vi "WHD_VEten_0.1.1_Pruebas.vi"() -> ()   [LabVIEW 2015]
uses:
  <vilib>/LabVIEW Targets/FPGA/cRIO/shared/nicrio_ModuleControls/nicrio_cRIO-9234_DataRatesRing2.ctl
  <vilib>/RTwatchdog.llb/Watchdog expiration actions.ctl
  <vilib>/userdefined/High Color/nirio_resource_hc.ctl
  <vilib>/FPGAPlugInAG/cRIO-9031/niLvFpga_Open_cRIO-9031.vi
  <vilib>/Utility/file.llb/Write Delimited Spreadsheet (string).vi
  <vilib>/FPGAPlugInAG/cRIO-9031/niLvFpga_Run_cRIO-9031.vi
  <vilib>/Utility/error.llb/Error Cluster From Error Code.vi
  <vilib>/rvi/errors/niLvFpgaAdjustHostInterfaceError.vi
  <vilib>/rvi/interface/common/niFpgaWaitOnOcc.vi
  <vilib>/FPGAPlugInAG/cRIO-9031/niLvFpga_Reset_cRIO-9031.vi
  <vilib>/FPGAPlugInAG/cRIO-9031/niLvFpga_Close_cRIO-9031.vi
  <vilib>/rvi/interface/nirviOpenFPGA/nirviOpenFPGA.xnode
  FPGA Bitfiles/W&RDEuskotrenIBA_FPGATarget2_FPGA8a2wsBIdirec_MwruJOs6jio.lvbitx
  <vilib>/rvi/interface/nirviMethod/nirviMethod.xnode
  <vilib>/rvi/interface/nirviReadWriteControl/nirviReadWriteControl.xnode
  <vilib>/rvi/interface/nirviCloseFPGA/nirviCloseFPGA.xnode
  <vilib>/NI_Real-Time Target Support.lvlib
  NiFpgaLv.dll
  <vilib>/rvi/errors/niLvFpgaMergeErrorWithErrorCode.vi
  <vilib>/nisyscfg/nisyscfg.lvlib
  <vilib>/FPGAPlugInAG/cRIO-9031/niLvFpga_ConfigureFifo_cRIO-9031.vi
  <vilib>/FPGAPlugInAG/cRIO-9031/niLvFpga_StartFifo_cRIO-9031.vi
  <vilib>/FPGAPlugInAG/cRIO-9031/niLvFpga_ReadFifo_cRIO-9031.vi
  <vilib>/FPGAPlugInAG/cRIO-9031/niLvFpga_StopFifo_cRIO-9031.vi
  AURA_Wheel/Json2Labv.lvlib
  AURA_Wheel/AuraWheelAPI/AuraWheel.lvlib
panel:
  in  "stop":bool
  out "Direccion 0?":bool
  out "Boton Adquirir?":bool
  out "RuedaDetectada2?":bool=TRUE
  out "RuedaDetectada1?":bool=TRUE
  in  "Timeout ruedas":dbl
  in  "Borrar archivos\nadquisicion con error":bool
  in  "Disable watchdog?":bool
  in  "Reset watchdog?":bool
  in  "Leer config RFID NEM":bool
  in  "bytes to read":i32
  in  "DeviceAddress":u8
  in  "timeout ms (60000)":i32
  in  "Max archivos":u32=2
  in  "Bytes libre despues de borrar":u32=2
  in  "Bytes min libre":u32=2
  in  "Nº de acelerómetros":i32
  in  "Nº inductivos":i32
  in  "Offset_rueda WS 1":fxp<+/-,24,-4>=0.004999998956918716 format="%.27g"
  out "TAGs_AURAwheel":string[][](array[string])
  out "Plataformas?":bool
  out "Nº Ejes":i32[](array[numeric])
  out "Nº UTs":i32
  out "it-read-LR6":i32[](array[numeric])
  out "it-LR6":i32
  out "RFID_LR6_Error":errorcluster
  out "Series_flota":string[](array[string])
  out "Tabla_flota":string[][](array[string])
  out "Puntos medios de las ventanas":dbl[][](array[numeric])
  out "configuration file path":path=path "c:/Parametros.cfg"
  in  "IP synchr":string
  out "data":cluster{"status":string}
  out "confRFID":path=path "c:/RFID/TAGS.csv"
  out "TAGS leidos":path=path "c:/RFID/TAGS.csv"
  in  "Use Aura?":bool
  in  "Parametros AuraWheel":string[](array[string])
  in  "Parámetros acelerómetros":dbl[](array[numeric])
  in  "Tiempo de adquisicion":dbl=10.0
  in  "Adquirir":bool
  out "Fin":bool
  out "Contador":i32=1
  out "Path TEST":path=path "c:/TEST"
  out "Fallo fotocelula":bool
  out "Path_Borrar":path=path "c:/Trenes"
  out "Longitud de la unidad":dbl
  out "Aviso no detección":string
  out "Time to Acquire Block (ms)":i32
  out "Distancia de acelerómetros":dbl[](array[numeric])
  out "Block Size":u32
  out "Distancias generales":dbl[](array[numeric])
  in  "Reset del controlador":bool
  in  "Configuración":bool
  in  "Parar la aplicación":bool
  out "RFID":bool=TRUE
  out "date/time string":string
  out "Timeout ruedas":bool
  out "Tiempo":dbl
  out "Inicio pasada":timestamp
  out "Ultimo TEST":timestamp
  out "Fuente":bool=TRUE
  out "Estado":string
  out "RFID_ID":refnum<k5>
  out "DC OK":string
  out "Aviso temperatura":string
  in  "Tab Control":T1(tab)=enum."Parámetros"
  out "V (m/s)":dbl
  out "Temperatura (ºC)":dbl
  out "Max RMS Ruedas":dbl[][](array[numeric])
  out "result":bool
  out "TAGs":string[](array[string])
  out "Parar":bool
  out "TAGs LR6":string[](array[string])
  out "TAGs HEX":string[](array[string])
  out "Waveform Graph":sgl[][](graph)
  out "Nombre de archivo":path[](array[path])
  out "Tiempo de paso (s)":dbl
  out "Tiempo extra de adquisición (s)":dbl
  out "Número de ejes detectados":i32
  out "Buffer Underflow":bool
  out "Buffer Overflow":bool
  out "created path":path
  out "Nº Ruedas 1":i32
  out "NºRuedas 2":i32
  out "deleted portion":sgl[](array[numeric])
  out "deleted portion 2":sgl[](array[numeric])
  out "Ejes_convoy":i32
  out "T fuera rango":bool
  in  "Frecuencia de muestreo (Hz)":dbl=25600.0
  in  "Escaneos de la FIFO por canal":u32=5000
  in  "Tiempo extra al detector de paso (s)":dbl=1.0
  in  "dt RMS":dbl=256.0
  in  "Frecuencia de muestreo y módulo CRIO":T2=2 items=["51.200 kS/s (NI 9234)"=1, "25.600 kS/s (NI 9234)"=2, "17.067 kS/s (NI 9234)"=3, "12.800 kS/s (NI 9234)"=4, "10.240 kS/s (NI 9234)"=5, "8.533 kS/s (NI 9234)"=6, "7.314 kS/s (NI 9234)"=7, "6.400 kS/s (NI 9234)"=8, "5.689 kS/s (NI 9234)"=9, "5.120 kS/s (NI 9234)"=10, "4.654 kS/s (NI 9234)"=11, "4.267 kS/s (NI 9234)"=12, "3.938 kS/s (NI 9234)"=13, "3.657 kS/s (NI 9234)"=14, "3.413 kS/s (NI 9234)"=15, "3.200 kS/s (NI 9234)"=16, "3.012 kS/s (NI 9234)"=17, "2.845 kS/s (NI 9234)"=18, "2.695 kS/s (NI 9234)"=19, "2.560 kS/s (NI 9234)"=20, "2.438 kS/s (NI 9234)"=21, "2.328 kS/s (NI 9234)"=22, "2.226 kS/s (NI 9234)"=23, "2.133 kS/s (NI 9234)"=24, "2.048 kS/s (NI 9234)"=25, "1.969 kS/s (NI 9234)"=26, "1.896 kS/s (NI 9234)"=27, "1.829 kS/s (NI 9234)"=28, "1.765 kS/s (NI 9234)"=29, "1.707 kS/s (NI 9234)"=30, "1.652 kS/s (NI 9234)"=31]
  in  "Puerto RFID":u16=2189
  in  "IP RFID":string="192.168.106.99"
  in  "Offset_rueda WS 2":fxp<+/-,24,-4>=0.004999998956918716 format="%.27g"
  in  "Count(mSec)":u32=2
  in  "LR6 IP address":string="192.168.106.94"
  in  "Port LR6":u16=2001
  in  "RFID NEM on?":bool
  in  "RFID LR6 on?":bool
  in  "Canal cero WS1?":bool
  in  "Canal cero WS2":bool
  out "Parámetros":bool=TRUE
  out "Distacias y medidas de dispositivos":bool=TRUE
  out "RFID_Error":errorcluster
  out "error FPGA":errorcluster
  out "error manipulacion archivos":errorcluster
  out "Unidades y ejes":bool=TRUE
  out "RFID":bool=TRUE
  out "error AURA":errorcluster
  out "Response headers":string
  in  "Array":path[](array[path])=[path "c:/Trenes_prueba/0207_2013-09-24_19-09-42_0.bin", path "c:/Trenes_prueba/0096_2013-10-30_18-13-14_0.bin", path "c:/Trenes_prueba/0001_2013-06-05_13-06-23_0.bin"]
  out "Numeric 3":i32
  in  "Digital?":bool=TRUE
  out "Bucle Espera":i32
  out "Watchdog config":T3={"reset"=FALSE, "occurrence"=FALSE, "trigger protocol"=enum."active high", "trigger line"=enum."none", "disable watchdog on VI exit"=TRUE}
  # "Funciona?"
  # "Última detección de unidad"
  # "Error!!"
  # "Estado de la memoria"
  # "Parámetros de muestreo"
  # "Parámetros de adquisición"
  # "Parámetros de procesado"
  # "Cambio Fecha y Hora"
  # "Cargar datos de configuración"
  # "Errores!!"
  # "WRD_MEX\nWRD_ZAR"
  # "0 tagMexInit\n1 tagMexFin\n\n0 tag1\n1 tag2"
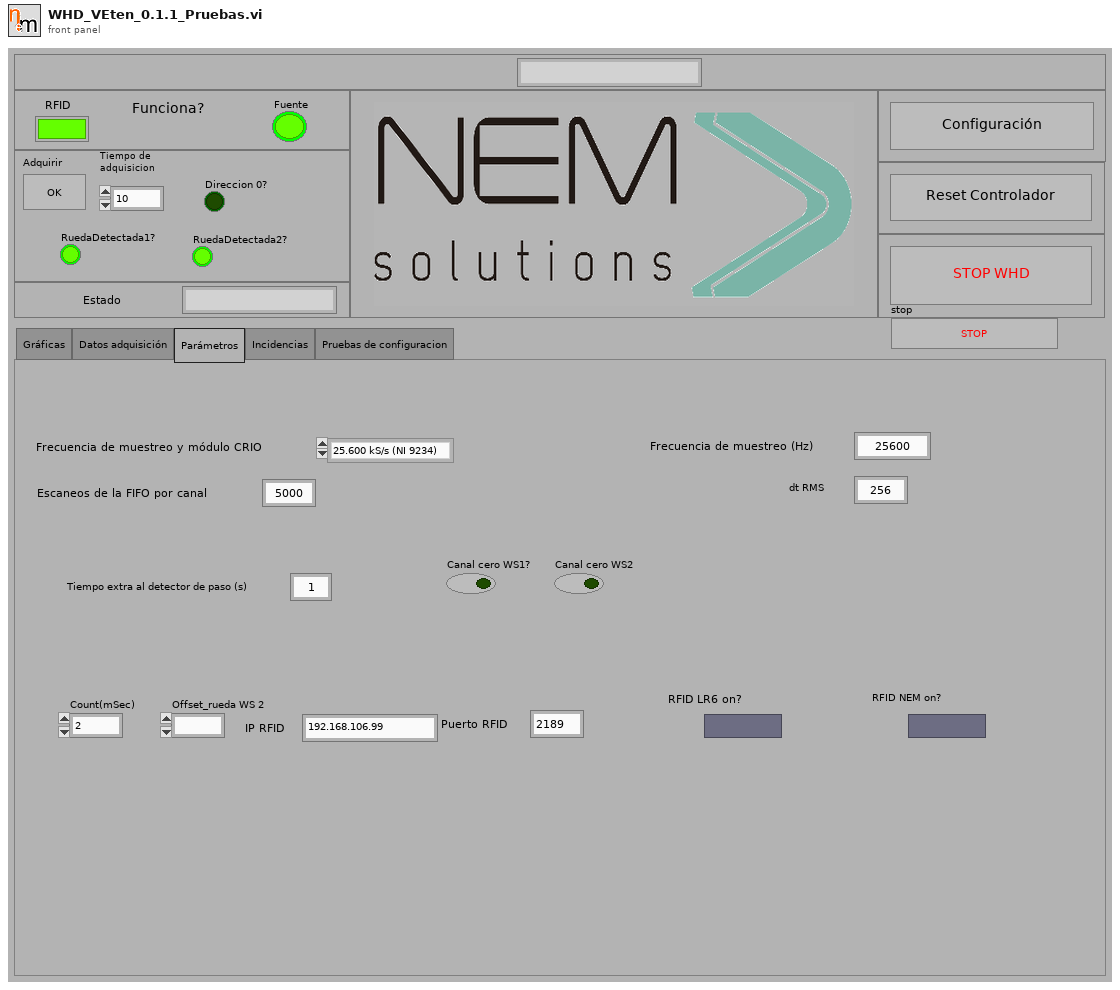
[diagram p1: front panel]
types:
  T1 = enum32{"Gráficas", "Datos adquisición", "Parámetros", "Incidencias", "Pruebas de configuracion"}
  T2 = typedef "nicrio_cRIO-9234_DataRatesRing2.ctl" = u8
  T3 = typedef "Watchdog expiration actions.ctl" = cluster{"reset":bool, "occurrence":bool, "trigger protocol":enum16{"active high", "active low", "open collector"}, "trigger line":enum16{"none", "line 0", "line 1", "line 2", "line 3", "line 4", "line 5", "line 6", "line 7", "SMB line 0"}, "disable watchdog on VI exit":bool}
  T4 = typedef "nirio_resource_hc.ctl" = tag
  T5 = enum16{"Standard", "Buffered", "CRLF", "Immediate"}
  T6 = enum16{"open", "replace", "create", "open or create", "replace or create", "replace or create with confirmation"}
  T7 = enum16{"big-endian, network order", "native, host order", "little-endian"}
  T8 = cluster{"error IO":errorcluster, bool[], u32[], string[], dbl[]}
  T9 = cluster{"g_ts":dbl, "p_sp":dbl, "p_tp":dbl, "p_tg":cluster{"tg_n":dbl, "tg_t":string}[], "p_ax":cluster{"ax_n":dbl, "ax_sp":dbl, "ax_wh":cluster{"wh_p":dbl, "wh_a1":dbl, "wh_a2":dbl, "wh_a3":dbl, "wh_a4":dbl}[]}[]}
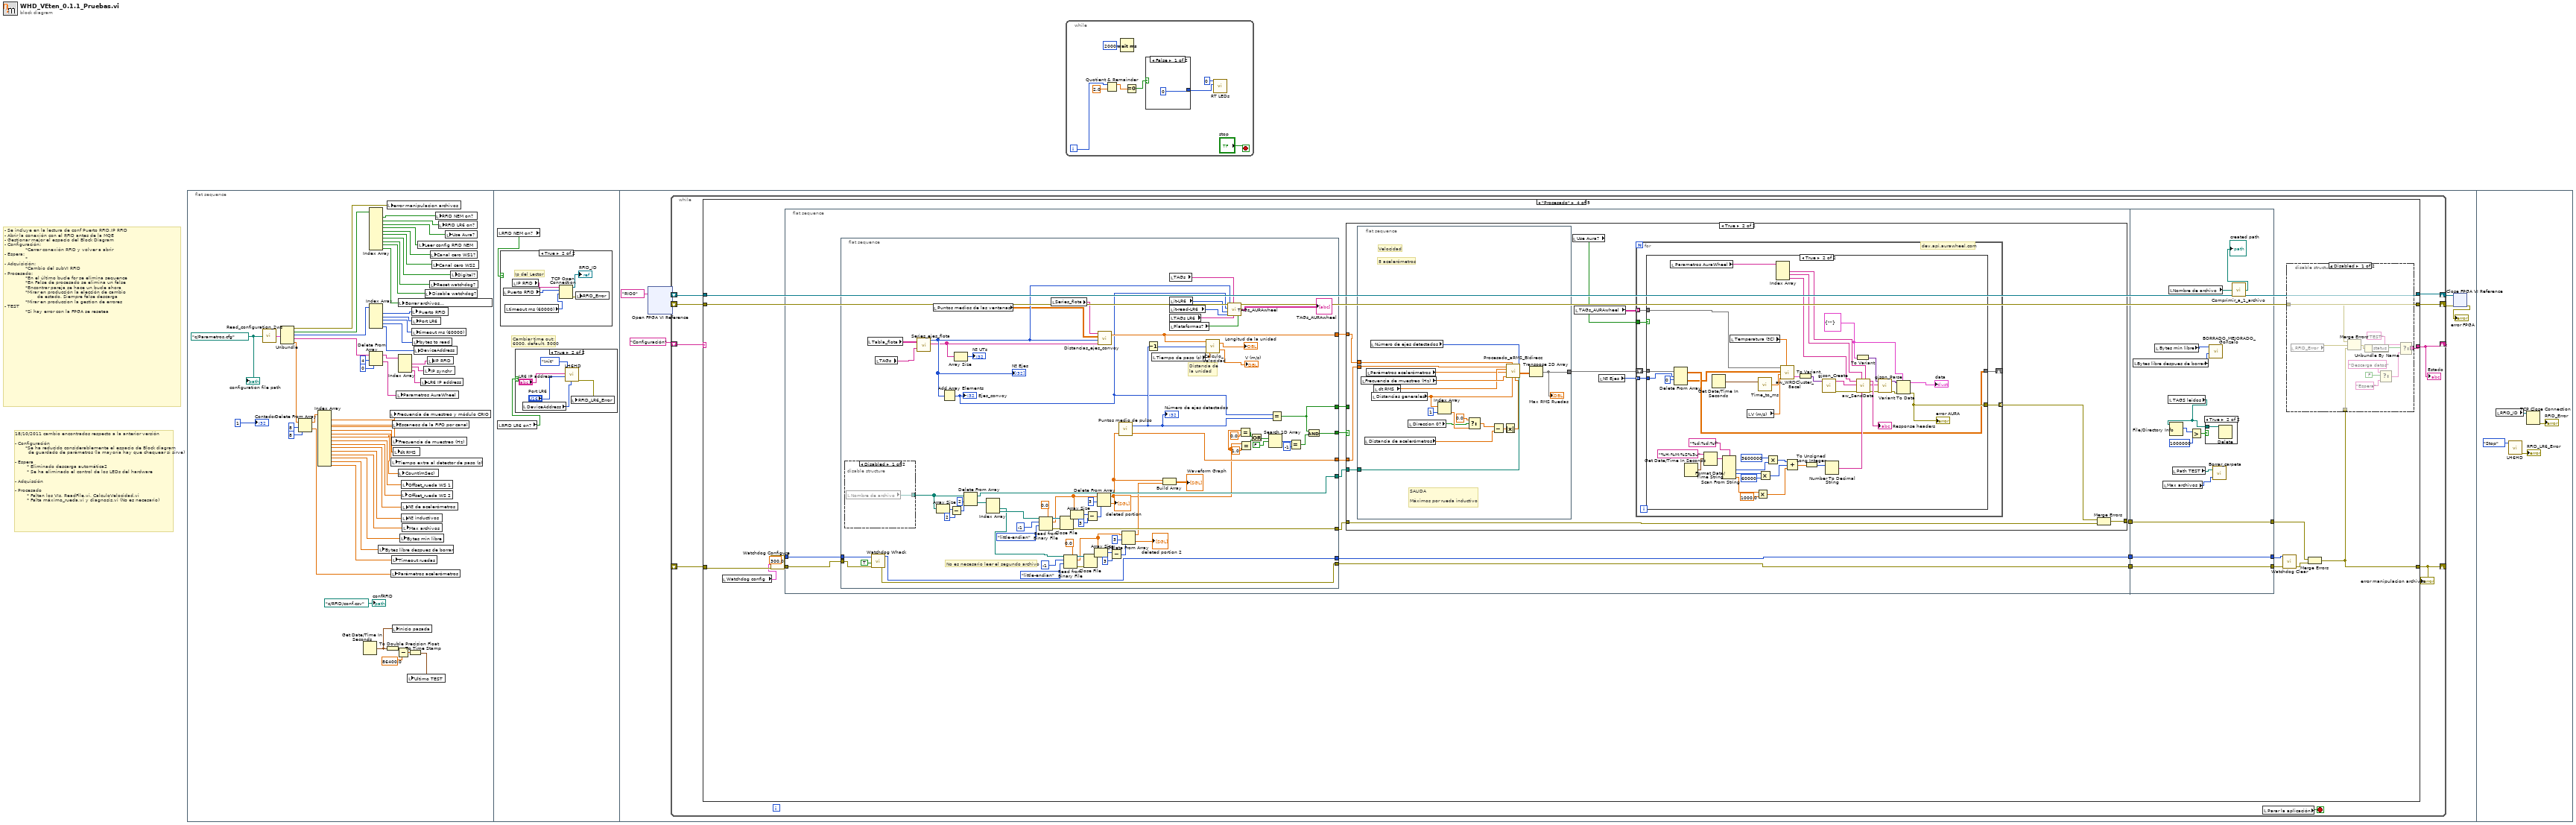
[diagram p0: block diagram]
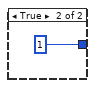
[diagram p2: hidden frame]
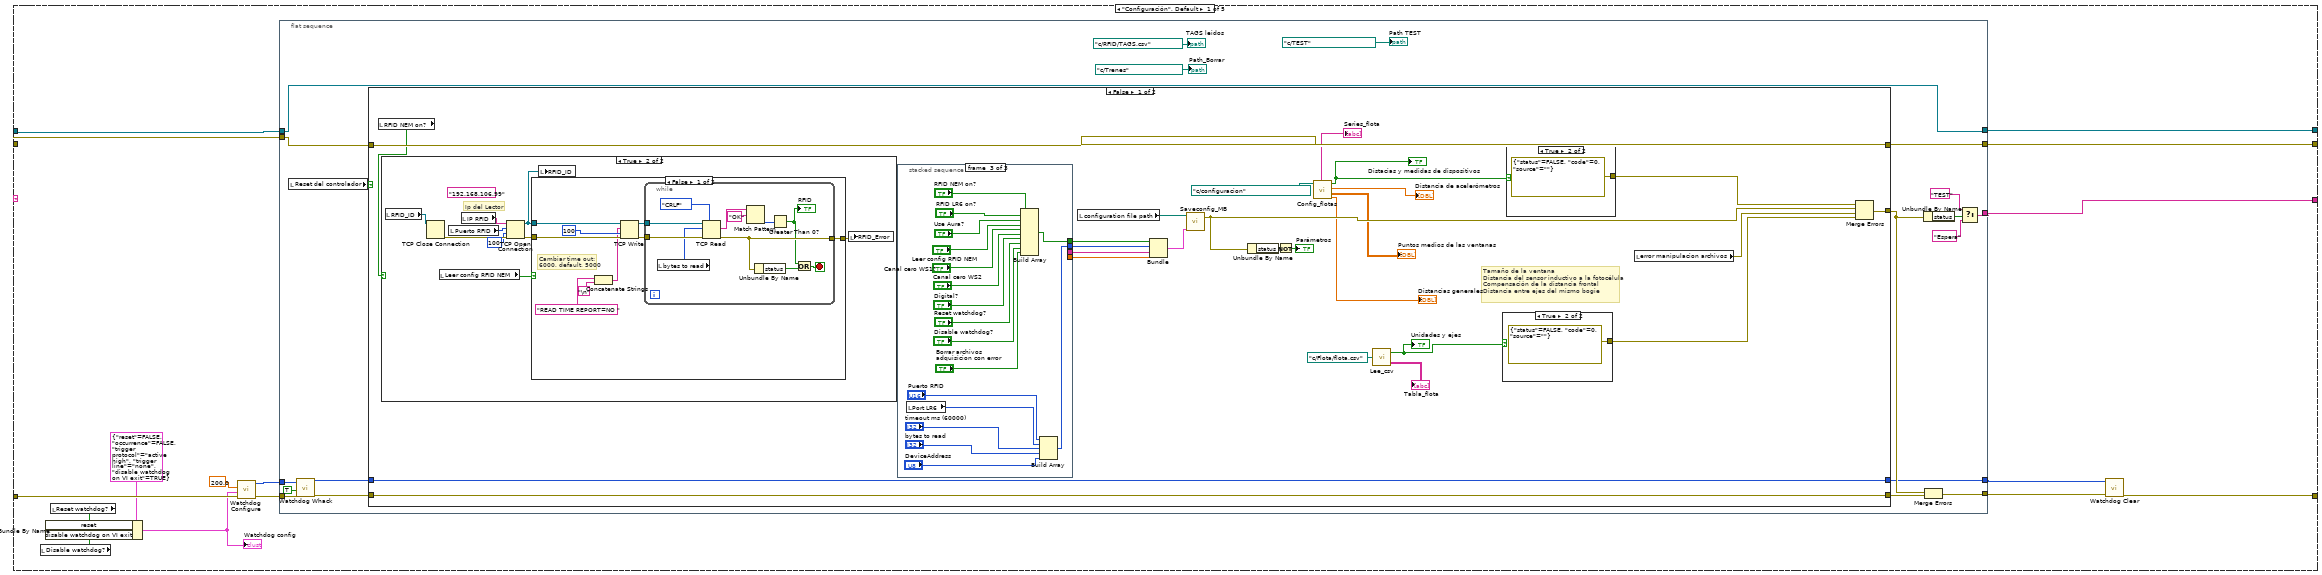
[diagram p5: hidden frame]
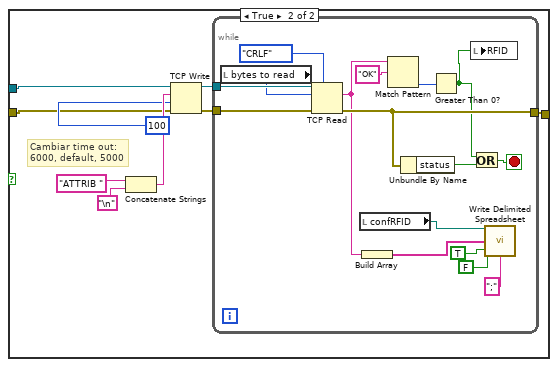
[diagram p7: hidden frame]
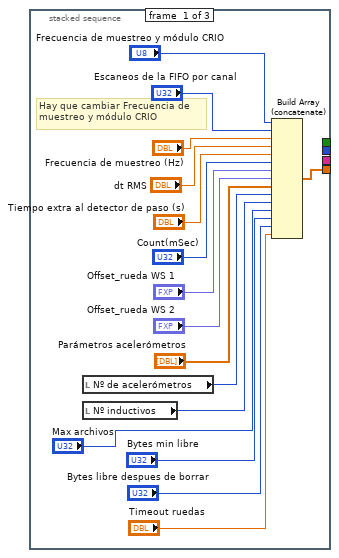
[diagram p8: hidden frame]
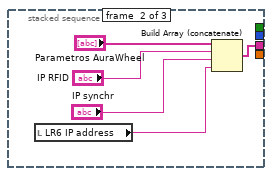
[diagram p9: hidden frame]
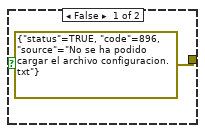
[diagram p10: hidden frame]
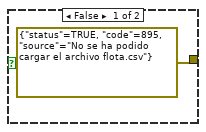
[diagram p11: hidden frame]
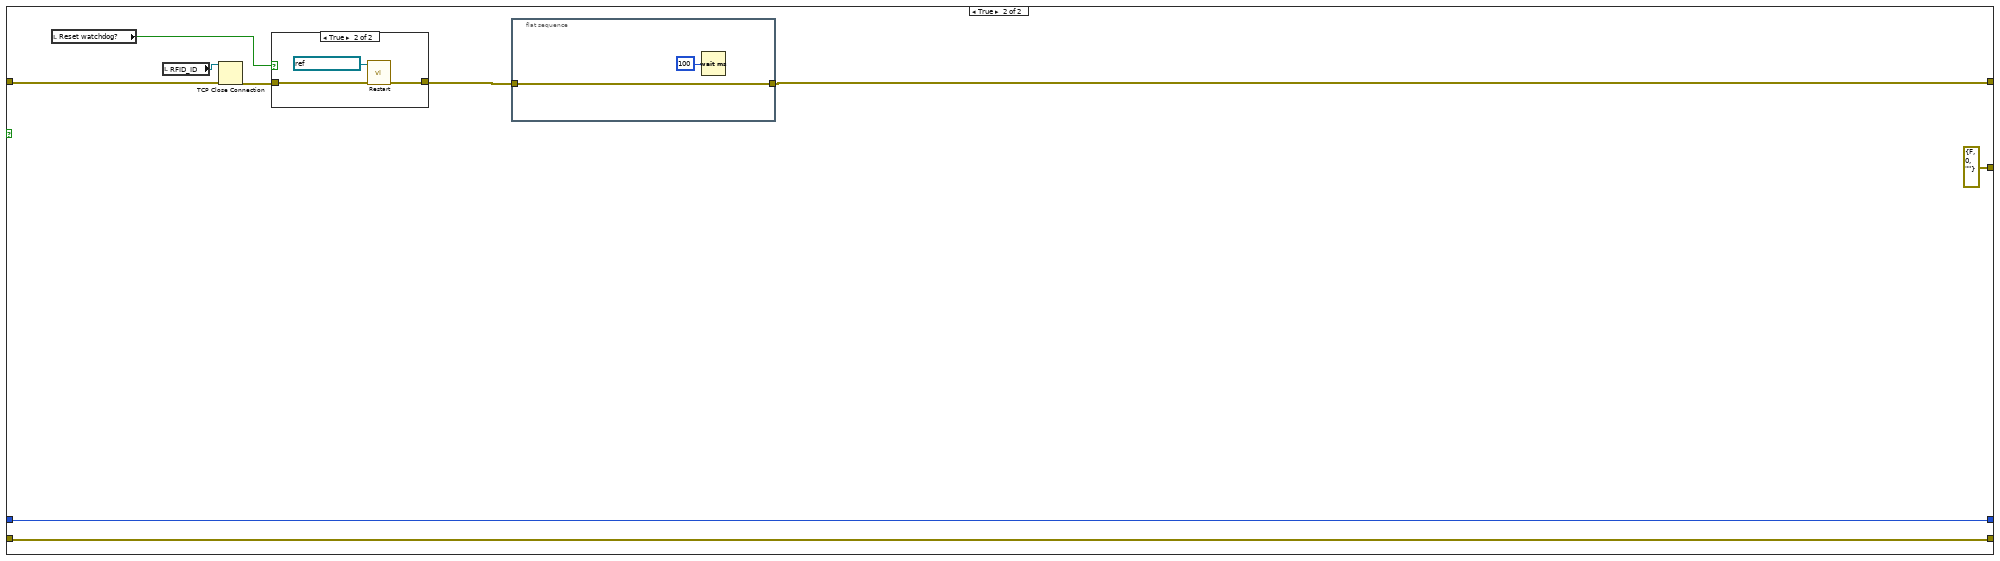
[diagram p12: hidden frame]
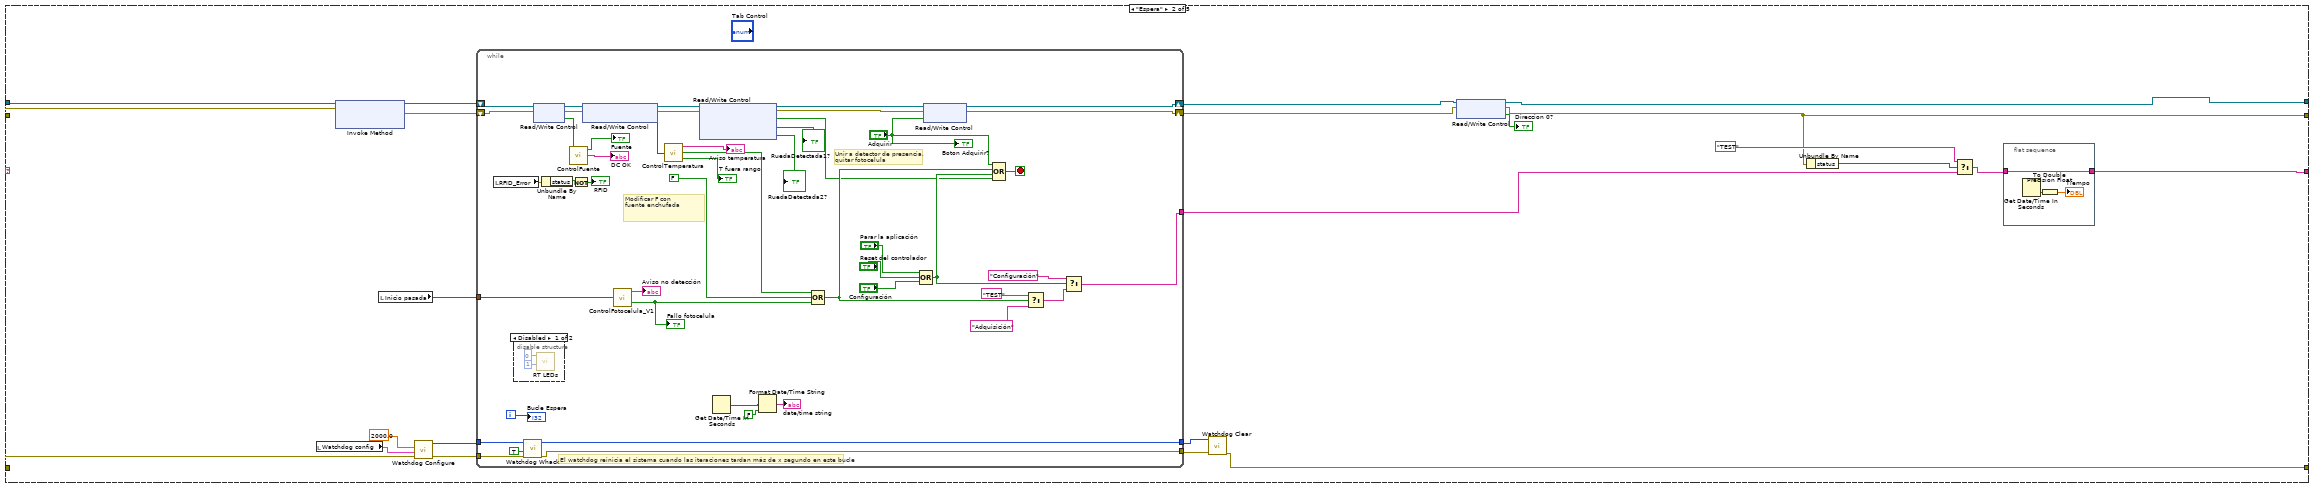
[diagram p14: hidden frame]
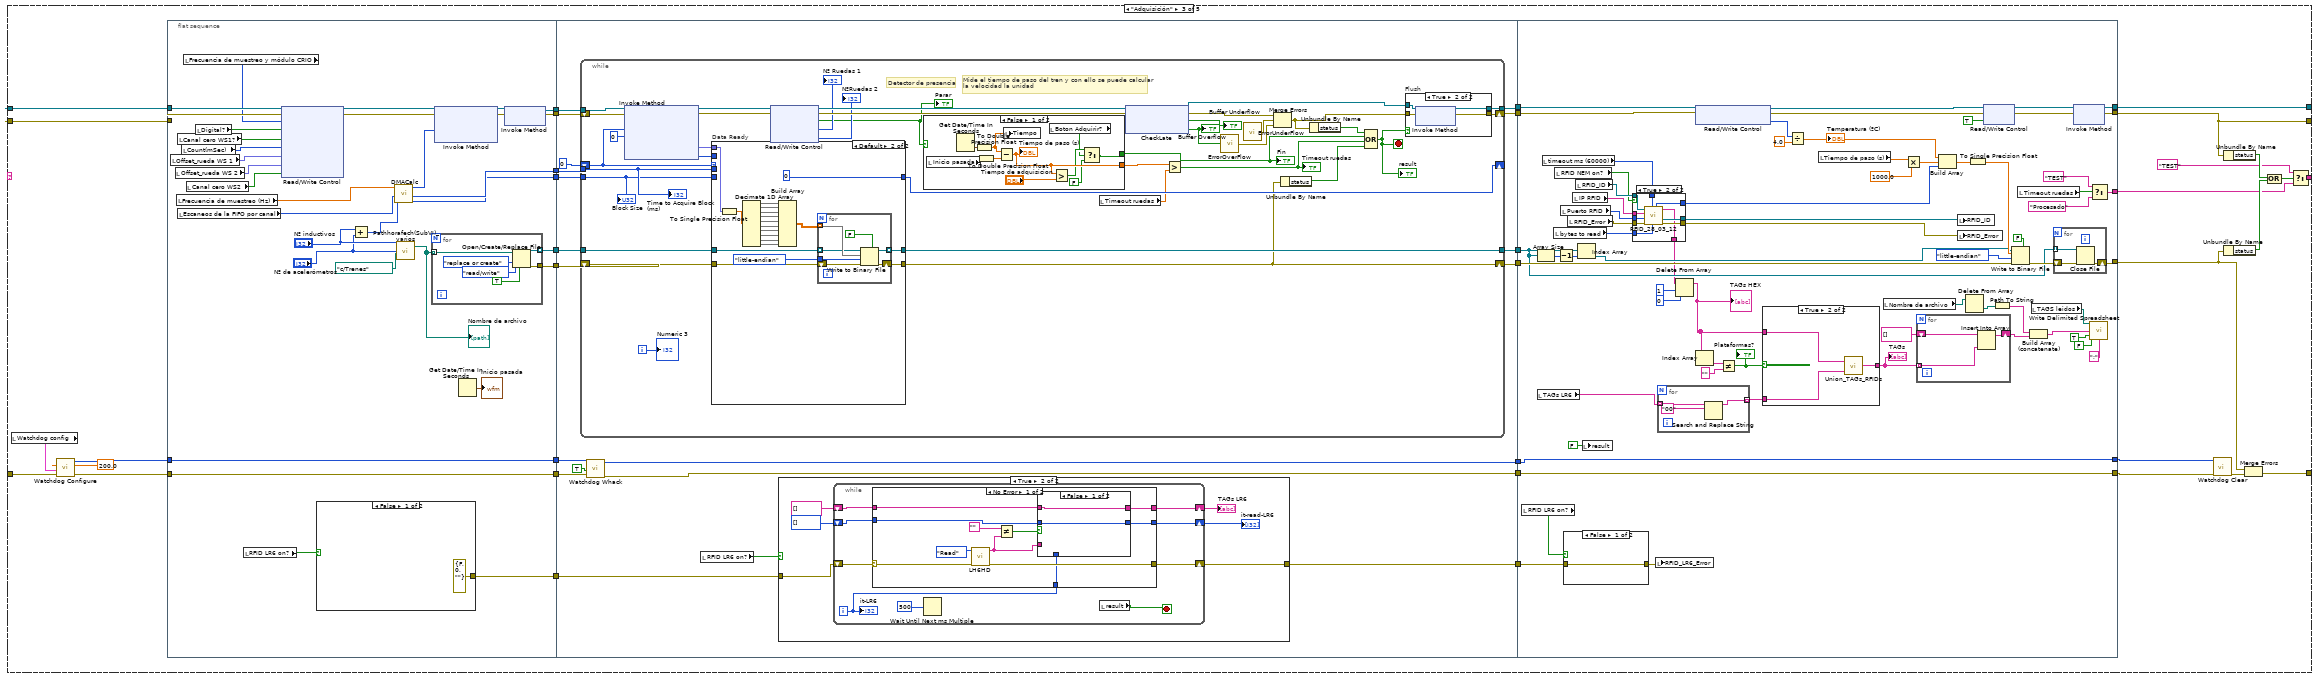
[diagram p16: hidden frame]
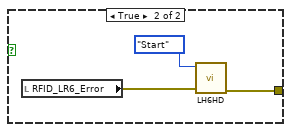
[diagram p17: hidden frame]
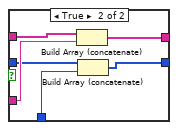
[diagram p19: hidden frame]
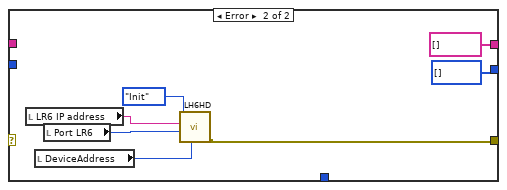
[diagram p20: hidden frame]
diagram:
  # "18/10/2011 cambio encontrados respecto a la anterior versión\n\n- Configuración\n       *Se ha reducido considerablemente el espacio de Block diagram\n         de guardado de parámetros (la mayoría hay que chequear si sirve)\n\n- Espera\n        * Eliminado descarga automática2\n        * Se ha eliminado el control de los LEDs del hardware\n       \n- Adquisción\n\n- Procesado\n        * Faltan los VIs, ReadFile.vi, CalculoVelocidad.vi\n        * Falta máximo_rueda.vi y diagnosis.vi (No es necesario)"
  # "- Se incluye en la lectura de conf Puerto RFID,IP RFID\n- Abrir la conexión con el RFID antes de la MQE\n- Gestionar mejor el espacio del Block Diagram\n- Configuración:\n              *Cerrar conexión RFID y volver a abrir\n- Espera:\n              *\n- Adquisición:\n              *Cambio del subVI RFID\n- Procesado:\n              *En el último bucle for se elimina sequence\n              *En False de procesado se elimina un false\n              *Encontrar pareja se hace un bucle ahora\n              *Mirar en producción la elección de cambio\n                      de estado. Siempre false descarga \n              *Mirar en produccion la gestion de errores\n- TEST\n              *Si hay error con la FPGA se resetea"
  n1 = flat-sequence {
    frame #0 {
      w38 = path "c:/Parametros.cfg" ("configuration file path")
      n2 = call "Read_configuration_2ws.vi"("configuration file path"=w38) -> ("output cluster"=w37:T8)
      n3 = Unbundle(w37) -> ("error IO"=w42:errorcluster, w41:bool[], w40:u32[], w29:string[], w35:dbl[])
      n4 = Delete From Array(array=w35, length=8, index=8) -> (deleted portion=w31:dbl[], array with subset deleted=w34:dbl[])
      n5 = Index Array(array=w34) -> (element #1=w49:dbl, element #2=w48:dbl, element #3=w47:dbl, element #4=w46:dbl, element #5=w45:dbl, element #6=w18:dbl, element #7=w17:dbl, element #8=w24:dbl, element #9=w16:dbl, element #10=w15:dbl, element #11=w14:dbl, element #12=w13:dbl, element #13=w12:dbl, element #14=w1:dbl)  [unwired: 14 in]
      n6 = Get Date/Time In Seconds() -> (seconds since 1Jan1904=w51:timestamp)
      n7 = Index Array(array=w41) -> (element #1=w44:bool, element #2=w43:bool, element #3=w30:bool, element #4=w8:bool, element #5=w7:bool, element #6=w6:bool, element #7=w5:bool, element #8=w4:bool, element #9=w3:bool, element #10=w2:bool)  [unwired: 10 in]
      n8 = Index Array(array=w40) -> (element #1=w36:u32, element #2=w19:u32, element #3=w11:u32, element #4=w10:u32, element #5=w9:u32)  [unwired: 5 in]
      n9 = Delete From Array(array=w29, length=4, index=0) -> (deleted portion=w22:string[], array with subset deleted=w28:string[])
      n10 = local write "Bytes libre despues de borrar"(w12) -> ()
      n11 = To Double Precision Float(number=w51) -> (double precision float=w53:dbl)
      n12 = local write "error manipulacion archivos"(w42) -> ()
      n13 = local write "Frecuencia de muestreo y módulo CRIO"(w49) -> ()
      n14 = local write "Parámetros acelerómetros"(w31) -> ()
      n15 = local write "Tiempo extra al detector de paso (s)"(w45) -> ()
      n16 = local write "Frecuencia de muestreo (Hz)"(w47) -> ()
      n17 = local write "Timeout ruedas"(w1) -> ()
      n18 = local write "Escaneos de la FIFO por canal"(w48) -> ()
      n19 = local write "Inicio pasada"(w51) -> ()
      n20 = local write "dt RMS"(w46) -> ()
      n21 = local write "Parametros AuraWheel"(w22) -> ()
      n22 = Subtract(x=w53, y=86400.0) -> (x-y=w52:dbl)
      n23 = local write "Borrar archivos\nadquisicion con error"(w2) -> ()
      n24 = Index Array(array=w28) -> (element #1=w21:string, element #2=w23:string, element #3=w20:string)  [unwired: 3 in]
      n25 = local write "Count(mSec)"(w18) -> ()
      n26 = local write "Bytes min libre"(w13) -> ()
      n27 = local write "Offset_rueda WS 2"(w24) -> ()
      n28 = local write "Offset_rueda WS 1"(w17) -> ()
      n29 = local write "Nº de acelerómetros"(w16) -> ()
      n30 = local write "Nº inductivos"(w15) -> ()
      n31 = local write "Max archivos"(w14) -> ()
      n32 = To Time Stamp(1:w52) -> (0:w50:timestamp)
      n33 = local write "Ultimo TEST"(w50) -> ()
      n34 = local write "Puerto RFID"(w36) -> ()
      n35 = local write "Port LR6"(w19) -> ()
      n36 = local write "timeout ms (60000)"(w11) -> ()
      n37 = local write "bytes to read"(w10) -> ()
      n38 = local write "DeviceAddress"(w9) -> ()
      n39 = local write "Leer config RFID NEM"(w8) -> ()
      n40 = local write "LR6 IP address"(w20) -> ()
      n41 = local write "IP synchr"(w23) -> ()
      n42 = local write "Disable watchdog?"(w3) -> ()
      n43 = local write "IP RFID"(w21) -> ()
      n44 = local write "Reset watchdog?"(w4) -> ()
      n45 = local write "Canal cero WS1?"(w7) -> ()
      n46 = local write "Canal cero WS2"(w6) -> ()
      n47 = local write "RFID NEM on?"(w44) -> ()
      n48 = local write "RFID LR6 on?"(w43) -> ()
      n49 = local write "Use Aura?"(w30) -> ()
      n50 = local write "Digital?"(w5) -> ()
      "Contador" <- 1
      "confRFID" <- path "c:/RFID/conf.csv" ("file path (use dialog)")
      "configuration file path" <- w38
    }
    frame #1 {
      # "Cambiar time out:\n6000, default, 5000"
      n51 = local read "RFID NEM on?"() -> (w56:bool)
      n52 = local read "RFID LR6 on?"() -> (w55:bool)
      n53 = case shown="True" w56 {
        frame False {
        }
        frame True {
          # "Ip del Lector"
          n54 = local read "Puerto RFID"() -> (w64:u16)
          n55 = local read "timeout ms (60000)"() -> (w62:i32)
          n56 = local read "IP RFID"() -> (w65:string)
          n57 = TCP Open Connection(address=w65, remote port or service name=w64, timeout ms (60000)=w62) -> (connection ID=→"RFID_ID":refnum<k5>, error out=w63:errorcluster)  [unwired: 1 in, 1 out]
          n58 = local write "RFID_Error"(w63) -> ()
        }
      }
      n59 = case shown="True" w55 {
        frame False {
        }
        frame True {
          n60 = local read "DeviceAddress"() -> (w57:u8)
          n61 = call "LH6HD.vi"("DeviceAddress"=w57, "Reader Port"="Port LR6", "IP Address"="LR6 IP address", "Action"=enum16{"Init", "Start", "Read", "Stop", "Exit"}."Init") -> ("error out"=w61:errorcluster)  [unwired: 6 in, 1 out]
          n62 = local write "RFID_LR6_Error"(w61) -> ()
        }
      }
    }
    frame #2 {
      n63 = xnode "Open FPGA VI Reference"("resource name"=T4 "RIO0") -> ("FPGA VI Reference Out"=w73:refnum<k20>, "error out"=w72:errorcluster)  [unwired: 1 in]
      n64 = while {
        shift-right: [w77] -> _
        shift-left: "Configuración" -> [w82]
        shift-right: [w75] -> w69
        shift-left: w73 -> [w81]
        shift-right: [w74] -> w68
        shift-left: w72 -> [w80]
        shift-right: [w79] -> _
        shift-left: _ -> [w78]
        stop <- w76 stop-if-true
        n65 = case shown="\"Procesado\"" w82 {
          tunnel: [w97 w269 w345 w677 w910] -> w77
          tunnel: [w96 w257 w359 w679 w909] -> w75
          tunnel: [w98 w256 w360 w674 w907] -> w74
          tunnel: w81 -> [w95 w274 w367 w679 w909]
          tunnel: w80 -> [w94 w272 w366 w674 w908]
          tunnel: [w87 w263 w357 w676 w897] -> w79
          tunnel: w78 -> [w93 w268 w341 w673 w902]
          frame "Configuración", Default {
            n66 = local read "Disable watchdog?"() -> (w85:bool)
            n67 = local read "Reset watchdog?"() -> (w84:bool)
            n68 = Bundle By Name(cluster=T3 {"reset"=FALSE, "occurrence"=FALSE, "trigger protocol"=enum."active high", "trigger line"=enum."none", "disable watchdog on VI exit"=TRUE} ("expiration actions"), "reset"=w84, "disable watchdog on VI exit"=w85) -> (w83:T3)
            "Watchdog config" <- w83
            n69 = call <vilib>:"Watchdog Configure.vi"("error in (no error)"=w93, "expiration actions"=w83, "timeout (1 sec)"=200.0) -> ("error out"=w90:errorcluster, "watchdogID"=w91:u64)  [unwired: 3 in, 2 out]
            n70 = flat-sequence {
              tunnel: [w109] -> w98
              tunnel: [w117] -> w97
              tunnel: w95 -> [w110]
              tunnel: [w110] -> w96
              tunnel: [w112] -> w88
              tunnel: w94 -> [w107]
              tunnel: w91 -> [w105]
              tunnel: w90 -> [w104]
              tunnel: [w102] -> w89
              frame #0 {
                n71 = local read "Reset del controlador"() -> (w106:bool)
                n72 = call <vilib>:"Watchdog Whack.vi"("error in (no error)"=w104, "reset watchdog after expire? (F)"=TRUE, "watchdogID in"=w105) -> ("error out"=w100:errorcluster, "watchdogID out"=w101:u64)  [unwired: 2 in, 1 out]
                n73 = case shown="False" w106 {
                  tunnel: w107 -> [w144 w247]
                  tunnel: [w144 w246] -> w109
                  tunnel: [w130 errorcluster {"status"=FALSE, "code"=0, "source"=""} ("error IO")] -> w108
                  tunnel: [w122 w245] -> w102
                  tunnel: w101 -> [w122 w245]
                  tunnel: w100 -> [w121 w244]
                  tunnel: [w121 w244] -> w99
                  frame False {
                    # "Tamaño de la ventana\nDistancia del sensor inductivo a la fotocélula\nCompensación de la distancia frontal\nDistancia entre ejes del mismo bogie"
                    n74 = local read "RFID NEM on?"() -> (w120:bool)
                    n75 = case shown="True" w120 {
                      frame False {
                      }
                      frame True {
                        (unwired) "192.168.106.99" ("address")
                        # "Ip del Lector"
                        n76 = local read "RFID_ID"() -> (w152:refnum<k5>)
                        n77 = TCP Close Connection(connection ID=w152) -> (error out=w153:errorcluster)  [unwired: 2 in, 1 out]
                        n78 = local read "Leer config RFID NEM"() -> (w145:bool)
                        n79 = local read "Puerto RFID"() -> (w150:u16)
                        n80 = local read "IP RFID"() -> (w149:string)
                        n81 = TCP Open Connection(address=w149, remote port or service name=w150, timeout ms (60000)=100, error in (no error)=w153) -> (connection ID=w151:refnum<k5>, error out=w146:errorcluster)  [unwired: 1 out]
                        n82 = case shown="False" w145 {
                          tunnel: w151 -> [w162 w176]
                          tunnel: [w160 w174] -> w147
                          tunnel: w146 -> [w157 w175]
                          frame False {
                            # "Cambiar time out:\n6000, default, 5000"
                            n83 = Concatenate Strings("READ TIME REPORT=NO " ("data in"), "\n") -> (w154:string)
                            n84 = TCP Write(connection ID=w162, data in=w154, error in (no error)=w157, 9:100 ("timeout ms (25000)")) -> (connection ID out=w158:refnum<k5>, error out=w159:errorcluster)  [unwired: 1 out]
                            n85 = while {
                              tunnel: w159 -> [w172]
                              tunnel: w158 -> [w171]
                              tunnel: [w170] -> w160
                              stop <- w167 stop-if-true
                              n86 = local read "bytes to read"() -> (w163:i32)
                              n87 = TCP Read(connection ID=w171, bytes to read=w163, error in (no error)=w172, 7:T5."CRLF" ("mode (standard)")) -> (data out=w165:string, error out=w170:errorcluster)  [unwired: 1 in, 1 out]
                              n88 = Match Pattern(string=w165, regular expression="OK") -> (offset past match=w168:i32)  [unwired: 4 out]
                              n89 = Unbundle By Name(w170) -> ("status"=w166:bool)
                              n90 = Greater Than 0?(x=w168) -> (x > 0?=w164:bool)
                              "RFID" <- w164
                              n91 = Or(x=w164, y=w166) -> (x .or. y?=w167:bool)
                            }
                          }
                          frame True {
                            # "Cambiar time out:\n6000, default, 5000"
                            n92 = Concatenate Strings("ATTRIB " ("data in"), "\n") -> (w182:string)
                            n93 = TCP Write(connection ID=w176, data in=w182, error in (no error)=w175, 9:100 ("timeout ms (25000)")) -> (connection ID out=w179:refnum<k5>, error out=w178:errorcluster)  [unwired: 1 out]
                            n94 = while {
                              tunnel: w178 -> [w197]
                              tunnel: w179 -> [w196]
                              tunnel: [w195] -> w174
                              stop <- w192 stop-if-true
                              n95 = local read "bytes to read"() -> (w183:i32)
                              n96 = TCP Read(connection ID=w196, bytes to read=w183, error in (no error)=w197, 7:T5."CRLF" ("mode (standard)")) -> (data out=w186:string, error out=w195:errorcluster)  [unwired: 1 in, 1 out]
                              n97 = local read "confRFID"() -> (w185:path)
                              n98 = Build Array(w186) -> (w184:string[])
                              n99 = Match Pattern(string=w186, regular expression="OK") -> (offset past match=w193:i32)  [unwired: 4 out]
                              n100 = Unbundle By Name(w195) -> ("status"=w191:bool)
                              n101 = Greater Than 0?(x=w193) -> (x > 0?=w190:bool)
                              n102 = local write "RFID"(w190) -> ()
                              n103 = Or(x=w190, y=w191) -> (x .or. y?=w192:bool)
                              n104 = call-poly <vilib>:"Write Delimited Spreadsheet.vi"("file path (dialog if empty)"=w185, "1D data"=w184, "append to file? (F)"=FALSE ("transpose? (no:F)"), "transpose? (F)"=TRUE ("append to file? (new file:F)"), "delimiter (\\t)"=";" ("delimiter (\\t)")) -> ()  [unwired: 9 in, 2 out]
                            }
                          }
                        }
                        n105 = local write "RFID_ID"(w151) -> ()
                        n106 = local write "RFID_Error"(w147) -> ()
                      }
                    }
                    n107 = stacked-sequence {
                      tunnel: [w210 _ _] -> w134
                      tunnel: [_ w219 _] -> w133
                      tunnel: [_ _ w233] -> w135
                      tunnel: [_ _ w232] -> w136
                      frame #0 {
                        # "Hay que cambiar Frecuencia de\nmuestreo y módulo CRIO"
                        n108 = local read "Nº de acelerómetros"() -> (w204:i32)
                        n109 = local read "Nº inductivos"() -> (w203:i32)
                        n110 = Build Array (concatenate)("Frecuencia de muestreo y módulo CRIO", "Escaneos de la FIFO por canal", "Frecuencia de muestreo (Hz)", "dt RMS", "Tiempo extra al detector de paso (s)", "Count(mSec)", "Offset_rueda WS 1", "Offset_rueda WS 2", "Parámetros acelerómetros", w204, w203, "Max archivos", "Bytes min libre", "Bytes libre despues de borrar", "Timeout ruedas") -> (w210:dbl[])
                      }
                      frame #1 {
                        n111 = local read "LR6 IP address"() -> (w215:string)
                        n112 = Build Array (concatenate)("Parametros AuraWheel", "IP RFID", "IP synchr", w215) -> (w219:string[])
                      }
                      frame #2 {
                        n113 = local read "Port LR6"() -> (w229:u16)
                        n114 = Build Array("RFID NEM on?", "RFID LR6 on?", "Use Aura?", "Leer config RFID NEM", "Canal cero WS1?", "Canal cero WS2", "Digital?", "Reset watchdog?", "Disable watchdog?", "Borrar archivos\nadquisicion con error") -> (w232:bool[])
                        n115 = Build Array("Puerto RFID", w229, "timeout ms (60000)", "bytes to read", "DeviceAddress") -> (w233:i32[])
                      }
                    }
                    n116 = local read "configuration file path"() -> (w131:path)
                    n117 = Bundle(w136, w135, w133, w134) -> (w132:cluster{bool[], i32[], string[], dbl[]})  [unwired: 1 in]
                    n118 = call "Saveconfig_MB.vi"("configuration file path"=w131, "Configuracion"=w132) -> ("error out"=w139:errorcluster)  [unwired: 4 in]
                    n119 = Unbundle By Name(w139) -> ("status"=w140:bool)
                    n120 = Not(x=w140) -> (.not. x?=→"Parámetros":bool)
                    n121 = call "Config_flotas.vi"("file path (dialog if empty)"=path "c:/configuracion") -> ("Distancias generales"=→"Distancias generales":dbl[], "Puntos medios de las ventanas"=→"Puntos medios de las ventanas":dbl[][], "Distancia de acelerómetros"=→"Distancia de acelerómetros":dbl[], "Distacias y medidas de dispositivos"=w129:bool, "Series_flota"=→"Series_flota":string[])  [unwired: 3 in]
                    "Distacias y medidas de dispositivos" <- w129
                    n122 = call "Lee_csv.vi"("Path"=path "c:/Flota/flota.csv") -> ("Tabla_flota"=→"Tabla_flota":string[][], "Lectura_OK?"=w126:bool)
                    "Unidades y ejes" <- w126
                    n123 = case shown="True" w126 {
                      tunnel: [errorcluster {"status"=TRUE, "code"=895, "source"="No se ha podido cargar el archivo flota.csv"} ("error out") errorcluster {"status"=FALSE, "code"=0, "source"=""} ("error out")] -> w137
                      frame False {
                      }
                      frame True {
                      }
                    }
                    n124 = case shown="True" w129 {
                      tunnel: [errorcluster {"status"=TRUE, "code"=896, "source"="No se ha podido cargar el archivo configuracion.txt"} ("error out") errorcluster {"status"=FALSE, "code"=0, "source"=""} ("error out")] -> w142
                      frame False {
                      }
                      frame True {
                      }
                    }
                    n125 = local read "error manipulacion archivos"() -> (w138:errorcluster)
                    n126 = Merge Errors(w142, w139, w138, w137) -> (w130:errorcluster)
                  }
                  frame True {
                    n127 = local read "Reset watchdog?"() -> (w241:bool)
                    n128 = local read "RFID_ID"() -> (w249:refnum<k5>)
                    n129 = TCP Close Connection(connection ID=w249, error in (no error)=w247) -> (error out=w243:errorcluster)  [unwired: 2 out]
                    n130 = case shown="True" w241 {
                      tunnel: w243 -> [w250 w253]
                      tunnel: [w250 w252] -> w242
                      frame False {
                      }
                      frame True {
                        n131 = call <vilib>:"Restart.vi"("error in (no error)"=w253, "Session in"=refnum<k21> "localhost") -> ("error out"=w252:errorcluster)  [unwired: 7 in, 2 out]
                      }
                    }
                    n132 = flat-sequence {
                      tunnel: [w255] -> w246
                      tunnel: w242 -> [w255]
                      frame #0 {
                        n133 = Wait (ms)(milliseconds to wait=u32 100) -> ()  [unwired: 1 out]
                      }
                    }
                  }
                }
                n134 = Unbundle By Name(w108) -> ("status"=w118:bool)
                n135 = Merge Errors(w108, w99) -> (w112:errorcluster)
                n136 = Select(t="TEST", s=w118, f="Espera") -> (s? t:f=w117:string)
                "Path_Borrar" <- path "c:/Trenes" ("file path (use dialog)")
                "Path TEST" <- path "c:/TEST" ("file path (use dialog)")
                "TAGS leidos" <- path "c:/RFID/TAGS.csv" ("file path (use dialog)")
              }
            }
            n137 = call <vilib>:"Watchdog Clear.vi"("error in (no error)"=w88, "watchdogID in"=w89) -> ("error out"=w87:errorcluster)  [unwired: 5 in]
          }
          frame "Espera" {
            n138 = local read "Watchdog config"() -> (w262:T3)
            n139 = xnode "Invoke Method"("FPGA VI Reference In"=w274, "error in"=w272) -> ("FPGA VI Reference Out"=w273:refnum<k20>, "error out"=w271:errorcluster)  [unwired: 1 in]
            n140 = local read "Inicio pasada"() -> (w278:timestamp)
            n141 = call <vilib>:"Watchdog Configure.vi"("error in (no error)"=w268, "expiration actions"=w262, "timeout (1 sec)"=2000.0) -> ("error out"=w267:errorcluster, "watchdogID"=w266:u64)  [unwired: 3 in, 2 out]
            n142 = while {
              tunnel: [w301] -> w277
              shift-right: [w289] -> w258
              shift-left: w273 -> [w303]
              shift-right: [w288] -> w259
              shift-left: w271 -> [w302]
              tunnel: w278 -> [w306]
              tunnel: w267 -> [w286]
              tunnel: w266 -> [w287]
              tunnel: [w285] -> w265
              tunnel: [w284] -> w264
              i -> [w282]
              stop <- w329 stop-if-true
              # "Modificar F con\nfuente enchufada"
              # "Unir a detector de presencia,\nquitar fotocelula"
              # "El watchdog reinicia el sistema cuando las iteraciones tardan más de x segundo en este bucle"
              n143 = local read "RFID_Error"() -> (w309:errorcluster)
              n144 = disable-structure shown="Disabled" {
                frame Disabled {
                  n145 = call <vilib>:"RT LEDs.vi"("State"=1, "LED Num"=0) -> ()  [unwired: 1 in, 5 out]
                }
                frame Enabled {
                }
              }
              n146 = call <vilib>:"Watchdog Whack.vi"("error in (no error)"=w286, "reset watchdog after expire? (F)"=TRUE, "watchdogID in"=w287) -> ("error out"=w284:errorcluster, "watchdogID out"=w285:u64)  [unwired: 2 in, 1 out]
              n147 = xnode "Read/Write Control"("FPGA VI Reference In"=w303, "error in"=w302) -> ("FPGA VI Reference Out"=w320:refnum<k20>, "error out"=w319:errorcluster, "DC OK"=w324:bool)
              n148 = Unbundle By Name(w309) -> ("status"=w307:bool)
              n149 = call "ControlFuente.vi"("DC OK 3"=w324) -> ("DC OK 2"=→"Fuente":bool, "DC OK"=→"DC OK":string)  [unwired: 1 out]
              n150 = Not(x=w307) -> (.not. x?=→"RFID":bool)
              n151 = xnode "Read/Write Control"("FPGA VI Reference In"=w320, "error in"=w319) -> ("FPGA VI Reference Out"=w315:refnum<k20>, "error out"=w314:errorcluster, "Chassis Temperature"=w322:i16)
              n152 = call "ControlFotocelula_V1.vi"("Tiempo de entrada a espera"=w306) -> ("Aviso no detección"=→"Aviso no detección":string, "Boolean"=w312:bool)
              "Fallo fotocelula" <- w312
              n153 = call "ControlTemperatura.vi"("Chassis Temperature"=w322) -> ("Aviso temperatura"=→"Aviso temperatura":string, "Boolean"=w316:bool, "T fuera rango"=→"T fuera rango":bool)
              n154 = xnode "Read/Write Control"("FPGA VI Reference In"=w315, "error in"=w314) -> ("FPGA VI Reference Out"=w305:refnum<k20>, "error out"=w304:errorcluster, "Detector de presencia"=w296:bool, "RuedaDetectada1?"=→"RuedaDetectada1?":bool, "RuedaDetectada2?"=→"RuedaDetectada2?":bool)
              n155 = Get Date/Time In Seconds() -> (seconds since 1Jan1904=w298:timestamp)
              n156 = Format Date/Time String(seconds (now)=w298, UTC format=FALSE) -> (date/time string=→"date/time string":string)  [unwired: 1 in]
              n157 = Compound Arithmetic op=OR(w316, FALSE ("value"), w312) -> (w313:bool)
              n158 = Compound Arithmetic op=OR("Parar la aplicación", "Reset del controlador", "Configuración") -> (w310:bool)
              n159 = xnode "Read/Write Control"("FPGA VI Reference In"=w305, "error in"=w304, "Fotocélula"="Adquirir") -> ("FPGA VI Reference Out"=w289:refnum<k20>, "error out"=w288:errorcluster)
              n160 = Compound Arithmetic op=OR("Adquirir", w313, w310, w296) -> (w329:bool)
              n161 = Select(t="TEST", s=w313, f="Adquisición") -> (s? t:f=w325:string)
              n162 = Select(t="Configuración", s=w310, f=w325) -> (s? t:f=w301:string)
              "Bucle Espera" <- w282
              "Boton Adquirir?" <- "Adquirir"
            }
            n163 = call <vilib>:"Watchdog Clear.vi"("error in (no error)"=w264, "watchdogID in"=w265) -> ("error out"=w263:errorcluster)  [unwired: 5 in]
            n164 = xnode "Read/Write Control"("FPGA VI Reference In"=w258, "error in"=w259) -> ("FPGA VI Reference Out"=w257:refnum<k20>, "error out"=w256:errorcluster, "Direccion 0?"=→"Direccion 0?":bool)
            n165 = Unbundle By Name(w256) -> ("status"=w276:bool)
            n166 = Select(t="TEST", s=w276, f=w277) -> (s? t:f=w270:string)
            n167 = flat-sequence {
              tunnel: [w280] -> w269
              tunnel: w270 -> [w280]
              frame #0 {
                n168 = Get Date/Time In Seconds() -> (seconds since 1Jan1904=w281:timestamp)
                n169 = To Double Precision Float(number=w281) -> (double precision float=→"Tiempo":dbl)
              }
            }
          }
          frame "Adquisición" {
            n170 = local read "Watchdog config"() -> (w342:T3)
            n171 = call <vilib>:"Watchdog Configure.vi"("error in (no error)"=w341, "expiration actions"=w342, "timeout (1 sec)"=200.0) -> ("error out"=w339:errorcluster, "watchdogID"=w340:u64)  [unwired: 3 in, 2 out]
            n172 = flat-sequence {
              tunnel: w366 -> [w395]
              tunnel: w367 -> [w396]
              tunnel: [w394] -> w356
              tunnel: [w393] -> w355
              tunnel: [w392] -> w354
              tunnel: [w391] -> w353
              tunnel: [w390] -> w352
              tunnel: [w389] -> w351
              tunnel: [w378] -> w344
              tunnel: w340 -> [w377]
              tunnel: w339 -> [w376]
              tunnel: [w377] -> w338
              tunnel: [w376] -> w337
              tunnel: [w411] -> w365
              tunnel: [w428] -> w364
              tunnel: [w427] -> w363
              tunnel: [w426] -> w362
              tunnel: [w419] -> w361
              tunnel: w356 -> [w425]
              tunnel: w355 -> [w424]
              tunnel: w354 -> [w423]
              tunnel: w353 -> [w422]
              tunnel: w352 -> [w421]
              tunnel: w351 -> [w420]
              tunnel: w344 -> [w417]
              tunnel: [w416] -> w343
              tunnel: w338 -> [w415]
              tunnel: w337 -> [w414]
              tunnel: [w412] -> w336
              tunnel: w365 -> [w579]
              tunnel: w364 -> [w570]
              tunnel: w363 -> [w569]
              tunnel: w362 -> [w595]
              tunnel: [w625] -> w348
              tunnel: w361 -> [w627]
              tunnel: [w611] -> w358
              tunnel: [w612] -> w360
              tunnel: [w613] -> w359
              tunnel: w343 -> [w589]
              tunnel: w336 -> [w580]
              tunnel: [w580] -> w334
              tunnel: [w579] -> w333
              frame #0 {
                n173 = local read "Offset_rueda WS 1"() -> (w369:fxp<+/-,24,-4>)
                n174 = local read "Offset_rueda WS 2"() -> (w370:fxp<+/-,24,-4>)
                n175 = local read "Frecuencia de muestreo (Hz)"() -> (w387:dbl)
                n176 = local read "Canal cero WS1?"() -> (w380:bool)
                n177 = local read "Escaneos de la FIFO por canal"() -> (w375:u32)
                n178 = local read "Count(mSec)"() -> (w379:u32)
                n179 = local read "Frecuencia de muestreo y módulo CRIO"() -> (w382:T2)
                n180 = local read "Canal cero WS2"() -> (w368:bool)
                n181 = local read "Digital?"() -> (w381:bool)
                n182 = local read "RFID LR6 on?"() -> (w371:bool)
                n183 = xnode "Read/Write Control"("FPGA VI Reference In"=w396, "error in"=w395, "Data Rate"=w382, "Digital?"=w381, "Canal cero WS1?"=w380, "Count(mSec)"=w379, "Offset_WS1"=w369, "Offset_WS2"=w370, "Canal cero WS2?"=w368) -> ("FPGA VI Reference Out"=w386:refnum<k20>, "error out"=w385:errorcluster)
                n184 = case shown="False" w371 {
                  tunnel: [errorcluster {"status"=FALSE, "code"=0, "source"=""} ("error out") w401] -> w378
                  frame False {
                  }
                  frame True {
                    n185 = local read "RFID_LR6_Error"() -> (w402:errorcluster)
                    n186 = call "LH6HD.vi"("error in (no error)"=w402, "Action"=enum16{"Init", "Start", "Read", "Stop", "Exit"}."Start") -> ("error out"=w401:errorcluster)  [unwired: 8 in, 1 out]
                  }
                }
                n187 = Add(x="Nº inductivos", y="Nº de acelerómetros") -> (x+y=w373:i32)
                n188 = call "DMACalc.vi"("Number of Channels"=w373, "Number of Samples"=w375, "Rate (Hz)"=w387) -> ("Block Size"=w391:u32, "Time to Acquire Block (ms)"=w392:i32, "Host Buffer Size"=w397:u32)  [unwired: 6 in]
                n189 = call "Pathhorafech(SubVI)_varios.vi"("Folder path"=path "c:/Trenes", "Nº de acelerómetros"="Nº de acelerómetros", "Nº inductivos"="Nº inductivos") -> ("Acel_Paths"=w383:path[])  [unwired: 1 in, 1 out]
                "Nombre de archivo" <- w383
                n190 = for {
                  tunnel: w383 -> [w406] mode=indexing
                  tunnel: [w405] -> w390 mode=indexing
                  tunnel: [w404] -> w389
                  n191 = Open/Create/Replace File(file path (use dialog)=w406, operation (0:open)=T6."replace or create", access (0:read/write)=enum16{"read/write", "read-only", "write-only"}."read/write", disable buffering (F)=TRUE) -> (refnum out=w405:refnum<file>, error out=w404:errorcluster)  [unwired: 1 in, 2 out]
                }
                n192 = xnode "Invoke Method"("FPGA VI Reference In"=w386, "error in"=w385, "Requested Depth"=w397) -> ("FPGA VI Reference Out"=w399:refnum<k20>, "error out"=w398:errorcluster)  [unwired: 1 out]
                n193 = Get Date/Time In Seconds() -> (seconds since 1Jan1904=→"Inicio pasada":timestamp)
                n194 = xnode "Invoke Method"("FPGA VI Reference In"=w399, "error in"=w398) -> ("FPGA VI Reference Out"=w394:refnum<k20>, "error out"=w393:errorcluster)
              }
              frame #1 {
                n195 = while "Data Acquisition" {
                  tunnel: w425 -> [w480]
                  shift-right: [w505] -> _
                  shift-left: u32 0 ("t") -> [w501]
                  tunnel: w423 -> [w506]
                  tunnel: w422 -> [w504]
                  shift-right: [w507] -> w427
                  shift-left: w424 -> [w498]
                  tunnel: [w502] -> w428
                  tunnel: w421 -> [w484]
                  tunnel: [w485] -> w426
                  shift-right: [w483] -> w419
                  shift-left: w420 -> [w494]
                  i -> [w479]
                  stop <- w503 stop-if-true
                  # "Detector de presencia"
                  # "Mide el tiempo de paso del tren y con ello se puede calcular\nla velocidad la unidad"
                  n196 = xnode "Invoke Method"("FPGA VI Reference In"=w480, "error in"=w498, "Number of Elements"=w501, "Timeout (ms)"=0) -> ("FPGA VI Reference Out"=w476:refnum<k20>, "error out"=w482:errorcluster, "Data"=w497:fxp<+/-,24,4>[], "Elements Remaining"=w499:u32)
                  n197 = case "Data Ready" shown="Default" w501 {
                    tunnel: w506 -> [w529 _]
                    tunnel: [w528 u32 0 ("t")] -> w505
                    tunnel: w504 -> [w530 _]
                    tunnel: w499 -> [w527 _]
                    tunnel: w497 -> [_ w552]
                    tunnel: w494 -> [w526 w551]
                    tunnel: [w526 w553] -> w483
                    tunnel: w484 -> [w525 w550]
                    tunnel: [w525 w549] -> w485
                    frame 0 {
                      # "En este caso se compara los elementos que quedan\nen la FIFO del controlador con el tamaño dell bloque\nque aparece en el panel frontal. Si el número de \nelementos en la FIFO es mayor o igual que el tamaño\n del bloque se pasa al siguiente caso y se guardan \nlos datos en un archivo. El reloj que aparece es una\nespera para no consumir recursos."
                      n198 = Greater Or Equal?(x=w527, y=w530) -> (x >= y?=w531:bool)
                      n199 = case shown="False" w531 {
                        tunnel: [u32 0 ("Block Size") w535] -> w528
                        tunnel: [w534 0 ("t")] -> w532
                        tunnel: w529 -> [w534 _]
                        tunnel: w530 -> [_ w535]
                        frame False {
                        }
                        frame True {
                        }
                      }
                      n200 = call "WaitMinTimeBetweenCall.vi"("Minimum ms between calls"=w532) -> ()  [unwired: 2 in]
                    }
                    frame Default {
                      n201 = To Single Precision Float(number=w552) -> (single precision float=w539:sgl[])
                      n202 = Decimate 1D Array(w539) -> (w545:sgl[], w548:sgl[], w547:sgl[], w546:sgl[], w544:sgl[], w543:sgl[], w542:sgl[], w541:sgl[], w540:sgl[], w537:sgl[])
                      n203 = Build Array(w545, w548, w547, w546, w544, w543, w542, w541, w540, w537) -> (w538:sgl[][])
                      n204 = for {
                        tunnel: T7."little-endian" ("byte order (0:big-endian, network order)") -> [w562]
                        shift-right: [w556] -> w553
                        shift-left: w551 -> [w557]
                        tunnel: w538 -> [w560] mode=indexing
                        tunnel: w550 -> [w559] mode=indexing
                        tunnel: [w558] -> w549 mode=indexing
                        n205 = Write to Binary File(file (use dialog)=w559, data=w560, error in=w557, 5:FALSE ("prepend array or string size? (T)"), 9:w562) -> (refnum out=w558:refnum<file>, error out=w556:errorcluster)  [unwired: 2 out]
                      }
                    }
                  }
                  n206 = xnode "Read/Write Control"("FPGA VI Reference In"=w476, "error in"=w482) -> ("FPGA VI Reference Out"=w496:refnum<k20>, "error out"=w495:errorcluster, "Parar"=w472:bool, "Nº Ruedas 1"=→"Nº Ruedas 1":i32, "NºRuedas 2"=→"NºRuedas 2":i32)
                  "Parar" <- w472
                  n207 = case shown="False" w472 {
                    tunnel: [w511 w520] -> w473
                    tunnel: [w513 0.0] -> w488
                    frame False {
                      n208 = local read "Inicio pasada"() -> (w516:timestamp)
                      n209 = Get Date/Time In Seconds() -> (seconds since 1Jan1904=w515:timestamp)
                      n210 = To Double Precision Float(number=w515) -> (double precision float=w514:dbl)
                      n211 = To Double Precision Float(number=w516) -> (double precision float=w517:dbl)
                      n212 = Subtract(x=w514, y=w517) -> (x-y=w513:dbl)
                      "Tiempo de paso (s)" <- w513
                      n213 = local write "Tiempo"(w514) -> ()
                      n214 = local read "Boton Adquirir?"() -> (w508:bool)
                      n215 = Greater?(x=w513, y="Tiempo de adquisicion") -> (0:w510:bool)
                      n216 = Select(t=w510, s=w508, f=FALSE) -> (s? t:f=w511:bool)
                    }
                    frame True {
                      n217 = local read "Tiempo"() -> (w524:dbl)
                      n218 = local read "Tiempo extra al detector de paso (s)"() -> (w519:dbl)
                      n219 = Get Date/Time In Seconds() -> (seconds since 1Jan1904=w521:timestamp)
                      n220 = To Double Precision Float(number=w521) -> (double precision float=w522:dbl)
                      n221 = Subtract(x=w522, y=w524) -> (x-y=w523:dbl)
                      "Tiempo extra de adquisición (s)" <- w523
                      n222 = Greater?(x=w523, y=w519) -> (0:w520:bool)
                    }
                  }
                  "Fin" <- w473
                  n223 = local read "Timeout ruedas"() -> (w471:dbl)
                  n224 = xnode ("CheckLate")("FPGA VI Reference In"=w496, "error in"=w495) -> ("FPGA VI Reference Out"=w478:refnum<k20>, "error out"=w491:errorcluster, "Buffer Underflow"=→"Buffer Underflow":bool, "Buffer Overflow"=w481:bool)
                  "Buffer Overflow" <- w481
                  n225 = Greater?(x=w488, y=w471) -> (0:w486:bool)
                  "Timeout ruedas" <- w486
                  n226 = call "ErrorOverFlow.vi"("Buffer Overflow"=w481) -> ("error out"=w489:errorcluster)
                  n227 = call "ErrorUnderFlow.vi"() -> ("error out"=w490:errorcluster)  [unwired: 1 in]
                  n228 = Merge Errors(w491, w490, w489) -> (w477:errorcluster)
                  n229 = Unbundle By Name(w483) -> ("status"=w487:bool)
                  n230 = Unbundle By Name(w477) -> ("status"=w493:bool)
                  n231 = Compound Arithmetic op=OR(w493, w473, w486, w487) -> (w503:bool)
                  "result" <- w503
                  n232 = case "Flush" shown="True" w503 {
                    tunnel: [w563 w568] -> w507
                    tunnel: [w564 w567] -> w502
                    tunnel: w478 -> [w564 w566]
                    tunnel: w477 -> [w563 w565]
                    frame False {
                    }
                    frame True {
                      n233 = xnode "Invoke Method"("FPGA VI Reference In"=w566, "error in"=w565) -> ("FPGA VI Reference Out"=w567:refnum<k20>, "error out"=w568:errorcluster)
                    }
                  }
                  "Block Size" <- w504
                  "Time to Acquire Block (ms)" <- w506
                  "Numeric 3" <- w479
                }
                n234 = call <vilib>:"Watchdog Whack.vi"("error in (no error)"=w414, "reset watchdog after expire? (F)"=TRUE, "watchdogID in"=w415) -> ("error out"=w411:errorcluster, "watchdogID out"=w412:u64)  [unwired: 2 in, 1 out]
                n235 = local read "RFID LR6 on?"() -> (w410:bool)
                n236 = case shown="True" w410 {
                  tunnel: w417 -> [w429 w435]
                  tunnel: [w429 w434] -> w416
                  frame False {
                  }
                  frame True {
                    n237 = while {
                      shift-right: [w442] -> w434
                      shift-left: w435 -> [w443]
                      shift-right: [w441] -> w432
                      shift-left: string[] [] -> [w440]
                      shift-right: [w436] -> w430
                      shift-left: i32[] [] -> [w437]
                      i -> [w438]
                      stop <- w439 stop-if-true
                      n238 = case shown="No Error" w443 {
                        selector: w443 -> [w454 _]
                        tunnel: [w453 w469] -> w442
                        tunnel: [w449 string[] []] -> w441
                        tunnel: w440 -> [w448 _]
                        tunnel: w438 -> [w447 _]
                        tunnel: w437 -> [w446 _]
                        tunnel: [w445 i32[] []] -> w436
                        frame No Error {
                          n239 = call "LH6HD.vi"("error in (no error)"=w454, "Action"=enum16{"Init", "Start", "Read", "Stop", "Exit"}."Read") -> ("error out"=w453:errorcluster, "Tag"=w450:string)  [unwired: 8 in]
                          n240 = Not Equal?(x="", y=w450) -> (x != y?=w451:bool)
                          n241 = case shown="False" w451 {
                            tunnel: w450 -> [_ w463]
                            tunnel: [w457 w462] -> w449
                            tunnel: w448 -> [w457 w461]
                            tunnel: w447 -> [_ w458]
                            tunnel: w446 -> [w456 w460]
                            tunnel: [w456 w459] -> w445
                            frame False {
                            }
                            frame True {
                              n242 = Build Array (concatenate)(w461, w463) -> (w462:string[])
                              n243 = Build Array (concatenate)(w460, w458) -> (w459:i32[])
                            }
                          }
                        }
                        frame Error {
                          n244 = local read "LR6 IP address"() -> (w466:string)
                          n245 = local read "DeviceAddress"() -> (w464:u8)
                          n246 = local read "Port LR6"() -> (w467:u16)
                          n247 = call "LH6HD.vi"("DeviceAddress"=w464, "Reader Port"=w467, "IP Address"=w466, "Action"=enum16{"Init", "Start", "Read", "Stop", "Exit"}."Init") -> ("error out"=w469:errorcluster)  [unwired: 6 in, 1 out]
                        }
                      }
                      n248 = Wait Until Next ms Multiple(millisecond multiple=u32 500) -> ()  [unwired: 1 out]
                      n249 = local read "result"() -> (w439:bool)
                      "it-LR6" <- w438
                    }
                    "TAGs LR6" <- w432
                    "it-read-LR6" <- w430
                  }
                }
              }
              frame #2 {
                n250 = local read "RFID LR6 on?"() -> (w571:bool)
                n251 = Array Size(array=w595) -> (size(s)=w593:i32)
                n252 = local read "TAGs LR6"() -> (w582:string[])
                n253 = local read "timeout ms (60000)"() -> (w578:i32)
                n254 = local read "bytes to read"() -> (w577:i32)
                n255 = local read "RFID NEM on?"() -> (w576:bool)
                n256 = Decrement(x=w593) -> (x-1=w594:i32)
                n257 = local read "Puerto RFID"() -> (w610:u16)
                n258 = case shown="False" w571 {
                  tunnel: w589 -> [w635 w637]
                  tunnel: [w635 w636] -> w588
                  frame False {
                  }
                  frame True {
                    n259 = call "LH6HD.vi"("error in (no error)"=w637, "Action"=enum16{"Init", "Start", "Read", "Stop", "Exit"}."Stop") -> ("error out"=w636:errorcluster)  [unwired: 8 in, 1 out]
                  }
                }
                n260 = local read "RFID_Error"() -> (w621:errorcluster)
                n261 = local read "IP RFID"() -> (w592:string)
                n262 = local read "RFID_ID"() -> (w620:refnum<k5>)
                n263 = Index Array(array=w595, index=w594) -> (element=w603:refnum<file>)
                n264 = local write "result"(FALSE ("result")) -> ()
                n265 = case shown="True" w576 {
                  tunnel: [_ w650] -> w622
                  tunnel: w621 -> [w640 w649]
                  tunnel: w620 -> [w639 w648]
                  tunnel: [w639 w647] -> w619
                  tunnel: [w640 w646] -> w614
                  tunnel: w610 -> [_ w645]
                  tunnel: w592 -> [_ w644]
                  tunnel: [_ w643] -> w575
                  tunnel: w578 -> [_ w642]
                  tunnel: w577 -> [_ w641]
                  frame False {
                  }
                  frame True {
                    n266 = call "RFID_28_03_12.vi"("BYTES TO READ"=w641, "TIMEOUT"=w642, "RFID_Error"=w649, "Puerto RFID"=w645, "IP RFID"=w644, "RFID ID"=w648) -> ("RFID Error"=w646:errorcluster, "connection ID out"=w647:refnum<k5>, "TAGs HEX"=w643:string[], "Unidad"=w650:u32)  [unwired: 1 in]
                  }
                }
                n267 = local write "RFID_LR6_Error"(w588) -> ()
                n268 = for {
                  tunnel: w582 -> [w653] mode=indexing
                  tunnel: [w651] -> w581 mode=indexing
                  n269 = Search and Replace String(input string=w653, search string="00") -> (result string=w651:string)  [unwired: 6 in, 3 out]
                }
                n270 = Delete From Array(array=w575, length=1, index=0) -> (array with subset deleted=w572:string[])  [unwired: 1 out]
                "TAGs HEX" <- w572
                n271 = xnode "Read/Write Control"("FPGA VI Reference In"=w570, "error in"=w569) -> ("FPGA VI Reference Out"=w624:refnum<k20>, "error out"=w623:errorcluster, "Chassis Temperature"=w633:i16)
                n272 = Index Array(array=w572) -> (element=w587:string)  [unwired: 1 in]
                n273 = Not Equal?(x=w587, y="" ("delimiter (\\t)")) -> (x != y?=w585:bool)
                "Plataformas?" <- w585
                n274 = case shown="True" w585 {
                  tunnel: w581 -> [w654 w655]
                  tunnel: [w654 w657] -> w590
                  tunnel: w572 -> [_ w656]
                  frame False {
                  }
                  frame True {
                    n275 = call "Union_TAGs_RFIDs.vi"("TAGs LR6"=w655, "TAGs HEX"=w656) -> ("TAGs"=w657:string[])
                  }
                }
                "TAGs" <- w590
                n276 = Divide(x=w633, y=4.0) -> (x/y=w634:dbl)
                "Temperatura (ºC)" <- w634
                n277 = local read "Tiempo de paso (s)"() -> (w617:dbl)
                n278 = local read "Nombre de archivo"() -> (w602:path[])
                n279 = Multiply(x=w617, y=1000.0) -> (x*y=w615:dbl)
                n280 = for {
                  shift-right: [w663] -> w608
                  shift-left: string[] [] -> [w662]
                  tunnel: w590 -> [w661] mode=indexing
                  n281 = Insert Into Array(array=w662, new element=w661) -> (w663:string[])  [unwired: 1 in]
                }
                n282 = Build Array(w634, w615, w622) -> (w628:dbl[])
                n283 = local write "RFID_ID"(w619) -> ()
                n284 = local write "RFID_Error"(w614) -> ()
                n285 = Delete From Array(array=w602) -> (deleted portion=w601:path)  [unwired: 2 in, 1 out]
                n286 = To Single Precision Float(number=w628) -> (single precision float=w631:sgl[])
                n287 = xnode "Read/Write Control"("FPGA VI Reference In"=w624, "error in"=w623, "Stop"=TRUE ("stop")) -> ("FPGA VI Reference Out"=w605:refnum<k20>, "error out"=w604:errorcluster)
                n288 = Path To String(path=w601) -> (string=w607:string)
                n289 = Write to Binary File(file (use dialog)=w603, data=w631, error in=w627, 5:FALSE ("prepend array or string size? (T)"), 9:T7."little-endian" ("byte order (0:big-endian, network order)")) -> (error out=w600:errorcluster)  [unwired: 3 out]
                n290 = local read "Timeout ruedas"() -> (w618:bool)
                n291 = Build Array (concatenate)(w607, w608) -> (w583:string[])
                n292 = local read "TAGS leidos"() -> (w596:path)
                n293 = for {
                  shift-right: [w660] -> w611
                  shift-left: w600 -> [w659]
                  tunnel: w595 -> [w658] mode=indexing
                  n294 = Close File(refnum=w658, error in=w659) -> (error out=w660:errorcluster)  [unwired: 1 out]
                }
                n295 = xnode "Invoke Method"("FPGA VI Reference In"=w605, "error in"=w604) -> ("FPGA VI Reference Out"=w613:refnum<k20>, "error out"=w612:errorcluster)
                n296 = call-poly <vilib>:"Write Delimited Spreadsheet.vi"("file path (dialog if empty)"=w596, "1D data"=w583, "append to file? (F)"=FALSE ("transpose? (no:F)"), "transpose? (F)"=TRUE ("append to file? (new file:F)"), "delimiter (\\t)"=";" ("delimiter (\\t)")) -> ()  [unwired: 9 in, 2 out]
                n297 = Select(t="TEST", s=w618, f="Procesado") -> (s? t:f=w625:string)
              }
            }
            n298 = call <vilib>:"Watchdog Clear.vi"("error in (no error)"=w333, "watchdogID in"=w334) -> ("error out"=w335:errorcluster)  [unwired: 5 in]
            n299 = Unbundle By Name(w360) -> ("status"=w349:bool)
            n300 = Unbundle By Name(w358) -> ("status"=w350:bool)
            n301 = Merge Errors(w358, w335) -> (w357:errorcluster)
            n302 = Compound Arithmetic op=OR(w349, w350) -> (w347:bool)
            n303 = Select(t="TEST", s=w347, f=w348) -> (s? t:f=w345:string)
          }
          frame "Procesado" {
            n304 = local read "Watchdog config"() -> (w670:T3)
            n305 = call <vilib>:"Watchdog Configure.vi"("error in (no error)"=w673, "expiration actions"=w670, "timeout (1 sec)"=300.0) -> ("error out"=w672:errorcluster, "watchdogID"=w669:u64)  [unwired: 3 in, 2 out]
            n306 = flat-sequence {
              tunnel: w672 -> [w700]
              tunnel: [w701] -> w675
              tunnel: w669 -> [w699]
              tunnel: [w698] -> w668
              tunnel: [w697] -> w667
              tunnel: [w895] -> w678
              tunnel: w675 -> [w895]
              tunnel: [w894] -> w666
              tunnel: w668 -> [w894]
              tunnel: [w893] -> w665
              tunnel: w667 -> [w893]
              frame #0 {
                n307 = flat-sequence {
                  tunnel: [w880] -> w696
                  tunnel: [w877] -> w695
                  tunnel: w700 -> [w873]
                  tunnel: [w879] -> w694
                  tunnel: [w876] -> w691
                  tunnel: [w878] -> w693
                  tunnel: [w875] -> w692
                  tunnel: w699 -> [w874]
                  tunnel: [w872] -> w698
                  tunnel: [w871] -> w697
                  frame #0 {
                    # "No es necesario leer el segundo archivo"
                    # "Distancia de\nla unidad"
                    n308 = disable-structure shown="Disabled" {
                      disable-tunnel: [w881 "Array"] -> w865
                      frame Disabled {
                        n309 = local read "Nombre de archivo"() -> (w881:path[])
                      }
                      frame Enabled {
                      }
                    }
                    n310 = local read "Tabla_flota"() -> (w862:string[][])
                    n311 = call <vilib>:"Watchdog Whack.vi"("error in (no error)"=w873, "reset watchdog after expire? (F)"=TRUE, "watchdogID in"=w874) -> ("error out"=w871:errorcluster, "watchdogID out"=w872:u64)  [unwired: 2 in, 1 out]
                    n312 = local read "TAGs"() -> (w860:string[])
                    n313 = call "Series_ejes_flota.vi"("Tabla_flota"=w862, "Tags"=w860) -> ("Nº Ejes"=w864:i32[], "Series del convoy"=w859:string[])  [unwired: 2 in, 1 out]
                    "Nº Ejes" <- w864
                    n314 = local read "Puntos medios de las ventanas"() -> (w863:dbl[][])
                    n315 = Array Size(array=w865) -> (size(s)=w844:i32)
                    n316 = Add Array Elements(numeric array=w864) -> (sum=w867:i32)
                    "Ejes_convoy" <- w867
                    n317 = Subtract(x=w844, y=2 ("length")) -> (x-y=w846:i32)
                    n318 = Array Size(array=w859) -> (size(s)=→"Nº UTs":i32)
                    n319 = Delete From Array(array=w865, length=2, index=w846) -> (deleted portion=w832:path[], array with subset deleted=w878:path[])
                    n320 = Index Array(array=w832) -> (element #1=w819:path, element #2=w820:path)  [unwired: 2 in]
                    n321 = Read from Binary File(5:sgl 0.0, 9:T7."little-endian" ("byte order (0:big-endian, network order)"), 10:-1 ("count (1)"), 11:w820) -> (0:w842:errorcluster, 2:w834:sgl[], 3:w843:refnum<file>)  [unwired: 1 in, 2 out]
                    n322 = local read "Series_flota"() -> (w861:string[])
                    n323 = Close File(refnum=w843, error in=w842) -> (error out=w879:errorcluster)  [unwired: 1 out]
                    n324 = Read from Binary File(5:sgl 0.0, 9:T7."little-endian" ("byte order (0:big-endian, network order)"), 10:-1 ("count (1)"), 11:w819) -> (0:w830:errorcluster, 2:w822:sgl[], 3:w831:refnum<file>)  [unwired: 1 in, 2 out]
                    n325 = Array Size(array=w834) -> (size(s)=w838:i32)
                    n326 = Close File(refnum=w831, error in=w830) -> ()  [unwired: 2 out]
                    n327 = Subtract(x=w838, y=3 ("length")) -> (x-y=w836:i32)
                    n328 = Array Size(array=w822) -> (size(s)=w826:i32)
                    n329 = Delete From Array(array=w834, length=3, index=w836) -> (deleted portion=→"deleted portion":sgl[], array with subset deleted=w810:sgl[])
                    n330 = call "Distancias_ejes_convoy.vi"("Series_flota1"=w859, "Ejes_UT"=w864, "Puntos medios de las ventanas"=w863, "Series_flota"=w861) -> ("Distancias_entre_ejes_convoy"=w877:dbl[])  [unwired: 1 in]
                    n331 = Subtract(x=w826, y=3 ("length")) -> (x-y=w824:i32)
                    n332 = call "Puntos medio de pulso.vi"("DI Inductivo"=w810) -> ("Puntos"=w880:sgl[], "Número de ejes"=w870:i32)  [unwired: 1 in]
                    "Número de ejes detectados" <- w870
                    n333 = Delete From Array(array=w822, length=3, index=w824) -> (deleted portion=→"deleted portion 2":sgl[], array with subset deleted=w869:sgl[])
                    n334 = Decrement(x=w870) -> (x-1=w857:i32)
                    n335 = local read "Tiempo de paso (s)"() -> (w856:dbl)
                    n336 = Build Array(w810, w869) -> (→"Waveform Graph":sgl[][])
                    n337 = local read "TAGs"() -> (w853:string[])
                    n338 = local read "it-LR6"() -> (w850:i32)
                    n339 = local read "it-read-LR6"() -> (w851:i32[])
                    n340 = local read "TAGs LR6"() -> (w852:string[])
                    n341 = local read "Plataformas?"() -> (w849:bool)
                    n342 = call "Calculo_Velocidad.vi"("Tiempo de paso (s)"=w856, "Ejes"=w857, "Puntos iniciales de las ventanas"=w877) -> ("V (m/s)"=→"V (m/s)":dbl, "Longitud de la unidad"=→"Longitud de la unidad":dbl)
                    n343 = call "TAGs_AURAwheel.vi"("Nº Ejes"=w864, "TAGs"=w853, "Ejes_convoy"=w867, "it-LR6"=w850, "TAGs LR6"=w852, "it-read-LR6"=w851, "Plataformas?"=w849) -> ("TAGS_AURA"=→"TAGs_AURAwheel":string[][])  [unwired: 1 in]
                    n344 = Equal?(x=w810, y=0.0) -> (x = y?=w814:bool[])
                    n345 = Equal?(x=w810, y=1.0) -> (x = y?=w815:bool[])
                    n346 = Or(x=w814, y=w815) -> (x .or. y?=w811:bool[])
                    n347 = Search 1D Array(1D array=w811, element=FALSE) -> (index of element=w817:i32)  [unwired: 1 in]
                    n348 = Equal?(x=w867, y=w870) -> (x = y?=w875:bool)
                    n349 = Equal?(x=w817, y=-1) -> (x = y?=w809:bool)
                    n350 = And(x=w875, y=w809) -> (x .and. y?=w876:bool)
                  }
                }
                n351 = case shown="True" w691 {
                  tunnel: w694 -> [w704 w735]
                  tunnel: [w704 w734] -> w701
                  tunnel: w696 -> [_ w739]
                  tunnel: w695 -> [_ w737]
                  tunnel: w693 -> [_ w738]
                  tunnel: w692 -> [w703 _]
                  frame False {
                    n352 = local read "Nombre de archivo"() -> (w702:path[])
                    n353 = for {
                      tunnel: w702 -> [w706] mode=indexing
                      tunnel: w703 -> [w705]
                      n354 = flat-sequence {
                        tunnel: w706 -> [w716]
                        tunnel: [w716] -> w709
                        tunnel: [w715] -> w708
                        tunnel: w705 -> [w714]
                        tunnel: w709 -> [w723]
                        tunnel: [w722] -> w707
                        tunnel: w708 -> [w722]
                        tunnel: w707 -> [w725]
                        frame #0 {
                          w715 = path "c:/Est_Adq.csv" ("file path (use dialog)")
                          n355 = Path To String(path=w716) -> (string=w717:string)
                          n356 = Select(t="Nº Ejes detectados WS diferente a Nº Ejes TAGs" ("delimiter (\\t)"), s=w714, f="La señal del inductivo no es digital" ("delimiter (\\t)")) -> (s? t:f=w711:string)
                          n357 = Build Array(w717, w711) -> (w710:string[])
                          n358 = call-poly <vilib>:"Write Delimited Spreadsheet.vi"("file path (dialog if empty)"=w715, "1D data"=w710, "append to file? (F)"=FALSE ("transpose? (no:F)"), "transpose? (F)"=TRUE ("append to file? (new file:F)"), "delimiter (\\t)"=";" ("delimiter (\\t)")) -> ()  [unwired: 9 in, 2 out]
                        }
                        frame #1 {
                          n359 = local read "Borrar archivos\nadquisicion con error"() -> (w721:bool)
                          n360 = case shown="True" w721 {
                            tunnel: w723 -> [_ w724]
                            frame False {
                            }
                            frame True {
                              n361 = Delete(path (use dialog)=w724) -> ()  [unwired: 1 in, 6 out]
                            }
                          }
                        }
                        frame #2 {
                          n362 = File/Directory Info(path=w725) -> (size=w728:i64)  [unwired: 1 in, 6 out]
                          n363 = Greater?(x=w728, y=i64 1000000) -> (0:w726:bool)
                          n364 = case shown="True" w726 {
                            tunnel: w725 -> [_ w729]
                            frame False {
                            }
                            frame True {
                              n365 = Delete(path (use dialog)=w729) -> ()  [unwired: 4 in, 3 out]
                            }
                          }
                        }
                      }
                    }
                  }
                  frame True {
                    n366 = flat-sequence {
                      tunnel: w739 -> [w807]
                      tunnel: w738 -> [w806]
                      tunnel: w737 -> [w808]
                      tunnel: [w805] -> w736
                      frame #0 {
                        # "SALIDA \n\nMáximos por rueda inductivo"
                        # "8 acelerómetros"
                        # "Velocidad"
                        n367 = local read "Frecuencia de muestreo (Hz)"() -> (w804:dbl)
                        n368 = local read "Distancia de acelerómetros"() -> (w794:dbl[])
                        n369 = local read "Parámetros acelerómetros"() -> (w801:dbl[])
                        n370 = local read "Número de ejes detectados"() -> (w800:i32)
                        n371 = local read "Distancias generales"() -> (w799:dbl[])
                        n372 = local read "dt RMS"() -> (w803:dbl)
                        n373 = local read "Direccion 0?"() -> (w791:bool)
                        n374 = Index Array(array=w799, index=1) -> (element=w797:dbl)
                        n375 = Select(t=0.0, s=w791, f=w797) -> (s? t:f=w795:dbl)
                        n376 = Subtract(x=w795, y=w794) -> (x-y=w793:dbl[])
                        n377 = Absolute Value(x=w793) -> (abs(x)=w792:dbl[])
                        n378 = call "Procesado_aRMS_BIdirecc.vi"("Paths_canales_aRMS"=w806, "Ejes Procesados"=w800, "Distancias\nacelerometros"=w792, "Distancias generales (m)"=w799, "Distancias centrales de las ruedas\n               configuración (m)"=w808, "Frecuencia de muestreo"=w804, "Parámetros acelerómetros"=w801, "dt RMS 2"=w803, "Puntos"=w807) -> ("Max RMS Ruedas"=w802:dbl[][])  [unwired: 2 in]
                        n379 = Transpose 2D Array(2D array=w802) -> (transposed array=w805:dbl[][])
                        "Max RMS Ruedas" <- w805
                      }
                    }
                    n380 = local read "Use Aura?"() -> (w732:bool)
                    n381 = local read "TAGs_AURAwheel"() -> (w731:string[][])
                    n382 = local read "Nº Ejes"() -> (w730:i32[])
                    n383 = for {
                      tunnel: w732 -> [w744]
                      tunnel: [w743] -> w733 mode=indexing
                      tunnel: w731 -> [w742] mode=indexing
                      shift-right: [w741] -> _
                      shift-left: w736 -> [w745]
                      tunnel: w730 -> [w740] mode=indexing
                      # "dev.api.aurawheel.com"
                      n384 = case shown="True" w744 {
                        tunnel: w745 -> [w746 w756]
                        tunnel: [errorcluster {"status"=FALSE, "code"=0, "source"=""} ("error out") w761] -> w743
                        tunnel: w742 -> [_ w757]
                        tunnel: [w746 w755] -> w741
                        tunnel: w740 -> [_ w753]
                        frame False {
                        }
                        frame True {
                          w765 = cluster{"status":string} {"status"=""}
                          n385 = local read "Parametros AuraWheel"() -> (w790:string[])
                          n386 = Delete From Array(array=w756, length=w753, index (row)=0) -> (deleted portion=w752:dbl[][], array with subset deleted=w755:dbl[][])  [unwired: 1 in]
                          n387 = Get Date/Time In Seconds() -> (seconds since 1Jan1904=w786:timestamp)
                          n388 = Format Date/Time String(time format string (%c)="%H:%M:%S%3u", seconds (now)=w786) -> (date/time string=w784:string)  [unwired: 1 in]
                          n389 = Get Date/Time In Seconds() -> (seconds since 1Jan1904=w760:timestamp)
                          n390 = Scan From String(format string="%d:%d:%f", input string=w784) -> (output 1=w781:i32, output 2=w780:i32, output 3=w778:dbl)  [unwired: 5 in, 3 out]
                          n391 = local read "Temperatura (ºC)"() -> (w758:dbl)
                          n392 = local read "V (m/s)"() -> (w748:dbl)
                          n393 = Multiply(x=w778, y=1000.0) -> (x*y=w774:dbl)
                          n394 = call "Time_to_ms.vi"("seconds since 1Jan1904"=w760) -> ("Numeric"=w759:dbl)  [unwired: 1 in]
                          n395 = Multiply(x=w780, y=60000) -> (x*y=w775:i32)
                          n396 = Multiply(x=3600000, y=w781) -> (x*y=w776:i32)
                          n397 = Index Array(array=w790) -> (element #1=w751:string, element #2=w750:string, element #3=w749:string)  [unwired: 3 in]
                          n398 = call "aw_WRDCluster_8acel.vi"("Array TAGs"=w757, "Max RMS Ruedas"=w752, "TimeStamp"=w759, "p_sp"=w748, "p_tp"=w758) -> ("JSON cluster"=w787:T9)  [unwired: 1 in]
                          n399 = Compound Arithmetic op=ADD(w776, w775, w774) -> (w773:dbl)
                          n400 = To Variant(anything=w787) -> (Variant=w770:variant)
                          n401 = To Unsigned Long Integer(number=w773) -> (unsigned 32bit integer=w772:u32)
                          n402 = call "gjson_Create.vi"("JSON Object in"=w770) -> ("error out"=w768:errorcluster, "JSON String Out"=w769:string)  [unwired: 9 in]
                          n403 = Number To Decimal String(number=w772) -> (decimal integer string=w771:string)  [unwired: 1 in]
                          n404 = To Variant(anything=w765) -> (Variant=w764:variant)
                          n405 = call "aw_SendData.vi"("pwd"=w751, "x-nem-datetime"=w771, "User"=w750, "error in"=w768, "JSON Object"=w769, "URL"=w749) -> ("error out"=w766:errorcluster, "Response JSON"=w767:string, "Response headers"=→"Response headers":string)  [unwired: 3 in]
                          n406 = call "gjson_Parse.vi"("error in"=w766, "JSON String In"=w767, "JSON Cluster"=w764) -> ("error out"=w762:errorcluster, "JSON Cluster Out"=w763:variant)  [unwired: 7 in]
                          n407 = Variant To Data(error in=w762, type=w765, Variant=w763) -> (data=→"data":cluster{"status":string}, error out=w761:errorcluster)
                          "error AURA" <- w761
                        }
                      }
                    }
                    n408 = Merge Errors(w733, w735) -> (w734:errorcluster)
                  }
                }
              }
              frame #1 {
                n409 = local read "Bytes libre despues de borrar"() -> (w884:u32)
                n410 = local read "Bytes min libre"() -> (w885:u32)
                n411 = local read "Max archivos"() -> (w886:u32)
                n412 = local read "TAGS leidos"() -> (w889:path)
                n413 = local read "Nombre de archivo"() -> (w887:path[])
                n414 = File/Directory Info(path=w889) -> (size=w892:i64)  [unwired: 1 in, 6 out]
                n415 = local read "Path TEST"() -> (w888:path)
                n416 = Greater?(x=w892, y=i64 1000000) -> (0:w890:bool)
                n417 = case shown="True" w890 {
                  tunnel: w889 -> [_ w896]
                  frame False {
                  }
                  frame True {
                    n418 = Delete(path (use dialog)=w896) -> ()  [unwired: 4 in, 3 out]
                  }
                }
                n419 = call "BORRADO_MEJORADO_Gonzalo.vi"("Bytes LIBRE OK"=w884, "Bytes Minimo de Memoria libre"=w885) -> ()  [unwired: 10 in]
                n420 = call "Borrar_carpeta.vi"("Nº Archivos Max"=w886, "Path Carpeta"=w888) -> ()  [unwired: 1 in]
                n421 = call "Comprimir_a_1_archivo.vi"("Acel_paths"=w887) -> ("path_Pasada"=→"created path":path)
              }
            }
            n422 = call <vilib>:"Watchdog Clear.vi"("error in (no error)"=w665, "watchdogID in"=w666) -> ("error out"=w664:errorcluster)  [unwired: 5 in]
            n423 = Merge Errors(w678, w664) -> (w676:errorcluster)
            n424 = disable-structure shown="Disabled" {
              disable-tunnel: [w684 _] -> w677
              disable-tunnel: w676 -> [w682 _]
              disable-tunnel: w674 -> [w680 _]
              frame Disabled {
                n425 = local read "RFID_Error"() -> (w681:errorcluster)
                n426 = Merge Errors(w680, w681, w682) -> (w690:errorcluster)
                n427 = Unbundle By Name(w690) -> ("status"=w685:bool)
                n428 = Select(t="Descarga datos", s=FALSE, f="Espera") -> (s? t:f=w687:string)
                n429 = Select(t="TEST", s=w685, f=w687) -> (s? t:f=w684:string)
              }
              frame Enabled {
              }
            }
          }
          frame "TEST" {
            n430 = local read "Watchdog config"() -> (w905:T3)
            n431 = call <vilib>:"Watchdog Configure.vi"("expiration actions"=w905, "timeout (1 sec)"=200.0) -> ("error out"=w906:errorcluster, "watchdogID"=w903:u64)  [unwired: 4 in, 2 out]
            n432 = flat-sequence {
              tunnel: [w921] -> w910
              tunnel: w906 -> [w916]
              tunnel: w908 -> [w935]
              tunnel: [w934] -> w898
              tunnel: [w917] -> w907
              tunnel: w903 -> [w915]
              tunnel: [w914] -> w901
              tunnel: w902 -> [w913]
              tunnel: [w912] -> w900
              frame #0 {
                n433 = call <vilib>:"Watchdog Whack.vi"("error in (no error)"=w916, "reset watchdog after expire? (F)"=TRUE, "watchdogID in"=w915) -> ("error out"=w912:errorcluster, "watchdogID out"=w914:u64)  [unwired: 2 in, 1 out]
                n434 = Get Date/Time In Seconds() -> (seconds since 1Jan1904=w928:timestamp)
                n435 = local read "Ultimo TEST"() -> (w929:timestamp)
                n436 = To Double Precision Float(number=w928) -> (double precision float=w930:dbl)
                n437 = Subtract(x=w930, y=3600.0) -> (x-y=w932:dbl)
                n438 = To Time Stamp(1:w932) -> (0:w933:timestamp)
                n439 = In Range and Coerce(upper limit=w928, x=w929, lower limit=w933) -> (In Range?=w927:bool)  [unwired: 1 out]
                n440 = case shown="False" w927 {
                  tunnel: w913 -> [w964 _]
                  tunnel: w935 -> [w940 w979]
                  tunnel: [w949 errorcluster {"status"=FALSE, "code"=0, "source"=""} ("error out")] -> w934
                  tunnel: [w940 w979] -> w917
                  frame False {
                    n441 = local read "Timeout ruedas"() -> (w941:bool)
                    n442 = local read "Aviso no detección"() -> (w947:string)
                    n443 = local read "Aviso temperatura"() -> (w946:string)
                    n444 = case shown="True" w941 {
                      selector: w941 -> [_ w976]
                      tunnel: ["\r" w977] -> w939
                      frame False {
                      }
                      frame True {
                        w966 = "\n"
                        n445 = local read "Nº Ruedas 1"() -> (w973:i32)
                        n446 = local read "NºRuedas 2"() -> (w968:i32)
                        n447 = call "ErrorRuedas.vi"("Buffer Overflow"=w976) -> ("error out"=w978:errorcluster)
                        n448 = Number To Decimal String(number=w973) -> (decimal integer string=w971:string)  [unwired: 1 in]
                        n449 = Number To Decimal String(number=w968) -> (decimal integer string=w967:string)  [unwired: 1 in]
                        n450 = Concatenate Strings("Error Wheel sensors", "\n", "WS1 (ruedas):", w971, w966, "WS2 (ruedas):", w967, w966) -> (w969:string)
                        n451 = call "Error.vi"("Error con..."=w969, "error comunicacion 2"=w978) -> ("String"=w977:string)
                      }
                    }
                    n452 = local read "RFID_Error"() -> (w943:errorcluster)
                    n453 = local read "RFID_LR6_Error"() -> (w937:errorcluster)
                    n454 = local read "DC OK"() -> (w945:string)
                    n455 = call "Cabecera.vi"() -> ("String"=w962:string)
                    n456 = call "Adquisicion.vi"("Aviso no detección"=w947) -> ("String"=w961:string)
                    n457 = call "Temperatura.vi"("Aviso temperatura"=w946) -> ("String"=w960:string)
                    n458 = call "Fuente.vi"("DC OK"=w945) -> ("String"=w959:string)
                    n459 = call "FPGA.vi"("error out"=w940) -> ("String"=w958:string)
                    n460 = call "Escritura.vi"("error out"=w964) -> ("String"=w957:string)
                    n461 = call "Error.vi"("Error con..."="Error con el lecto RFID NEM", "error comunicacion 2"=w943) -> ("String"=w942:string)
                    n462 = call "Error.vi"("Error con..."="Error con el lecto RFID LR6-HD", "error comunicacion 2"=w937) -> ("String"=w936:string)
                    n463 = Concatenate Strings(w962, w961, w960, w959, w958, w957, w942, w936, w939) -> (w963:string)
                    n464 = call "STRINGhorafechA(SubVI).vi"() -> ("STRINGhora_fecha"=w956:string)
                    n465 = Concatenate Strings(w956, ".txt" ("string")) -> (w952:string)
                    n466 = Get Date/Time In Seconds() -> (seconds since 1Jan1904=→"Ultimo TEST":timestamp)
                    n467 = Build Array("c", "TEST" ("element"), w952) -> (w954:string[])
                    n468 = Array of Strings to Path(0:w954) -> (2:w950:path)  [unwired: 1 out]
                    n469 = Write to Text File(file (use dialog)=w950, text=w963) -> (error out=w949:errorcluster)  [unwired: 1 in, 3 out]
                  }
                  frame True {
                  }
                }
                n470 = local read "Fallo fotocelula"() -> (w920:bool)
                n471 = Unbundle By Name(w917) -> ("status"=w918:bool)
                n472 = local read "T fuera rango"() -> (w926:bool)
                n473 = Compound Arithmetic op=OR(w918, w920) -> (w919:bool)
                n474 = local write "Reset del controlador"(w919) -> ()
                n475 = Select(t="Escape", s=w926, f="Espera") -> (s? t:f=w923:string)
                n476 = Select(t="Configuracion", s=w919, f=w923) -> (s? t:f=w921:string)
              }
            }
            n477 = call <vilib>:"Watchdog Clear.vi"("error in (no error)"=w900, "watchdogID in"=w901) -> ("error out"=w899:errorcluster)  [unwired: 5 in]
            n478 = Merge Errors(w899, w898) -> (w897:errorcluster)
          }
        }
        "Estado" <- w77
        "error manipulacion archivos" <- w79
        n479 = local read "Parar la aplicación"() -> (w76:bool)
      }
      n480 = xnode "Close FPGA VI Reference"("FPGA VI Reference In"=w69, "error in"=w68) -> ("error out"=→"error FPGA":errorcluster)
    }
    frame #3 {
      n481 = local read "RFID_ID"() -> (w983:refnum<k5>)
      n482 = call "LH6HD.vi"("Action"=enum16{"Init", "Start", "Read", "Stop", "Exit"}."Stop") -> ("error out"=→"RFID_LR6_Error":errorcluster)  [unwired: 9 in, 1 out]
      n483 = TCP Close Connection(connection ID=w983) -> (error out=→"RFID_Error":errorcluster)  [unwired: 1 in, 2 out]
    }
  }
  n484 = while {
    i -> [w989]
    stop <- "stop" stop-if-true
    n485 = Quotient & Remainder(x=w989, y=2.0) -> (x-y*floor(x/y)=w985:dbl)  [unwired: 1 out]
    n486 = Wait (ms)(milliseconds to wait=u32 2000) -> ()  [unwired: 1 out]
    n487 = Equal To 0?(x=w985) -> (x = 0?=w988:bool)
    n488 = case shown="False" w988 {
      tunnel: [0 ("LED Num") 1 ("State")] -> w987
      frame False {
      }
      frame True {
      }
    }
    n489 = call <vilib>:"RT LEDs.vi"("State"=w987, "LED Num"=0) -> ()  [unwired: 1 in, 5 out]
  }
